vi "Periodic Tasks.vi"(8 "error in":errorcluster) -> ()   [LabVIEW 2018]
doc: "This VI runs in parallel to other tasks. It can contain as many user-defined periodic loops as you need. These can carry out PID or other sorts of timed response."
uses:
  <vilib>/Rock Robotics/WPI/ThirdParty/Phoenix-LabVIEW/Motor Controller/Controls/CTRE_Phoenix_MotorControl_ControlMode.ctl
  <vilib>/Rock Robotics/WPI/Utilities/WPI_GetSetVariantRefNum.vi
  <vilib>/Rock Robotics/Network Tables/NT Write Boolean Array.vi
  <vilib>/Rock Robotics/Network Tables/NT Write Numeric Array.vi
  <vilib>/Rock Robotics/Network Tables/NT Write Boolean.vi
  <vilib>/Rock Robotics/WPI/RobotDrive/WPI_RobotDriveMecanumDrive_Cartesian.vi
  <vilib>/Rock Robotics/WPI/ThirdParty/Phoenix-LabVIEW/Motor Controller/Get/CTRE_Phoenix_MotorController_GetAnalogData.vi
  <vilib>/Rock Robotics/Network Tables/NT Write Number.vi
panel:
  in  "Jack speed 3-2":dbl=-1.0
  in  "Jack drive 1-2":dbl=-0.75
  in  "Jack speed 2-2":dbl=1.0
  in  "Jack speed 1-2":dbl=1.0
  in  "Arm speed-2":dbl=-0.41
  in  "Pre Climb 2":i32=146
  in  "Load Cargo":i32=385
  in  "Arm speed":dbl=-0.55
  in  "Jack speed 1":dbl=1.0
  in  "Jack speed 2":dbl=1.0
  in  "Jack drive 1":dbl=-0.75
  in  "Jack speed 3":dbl=-1.0
  in  "Pre Climb":i32=80
  in  "Release Time":i32=7
  in  "Grab Drive Time":i32=7
  in  "Grab Wait Time":i32=2
  in  "Grab Time":i32=5
  in  "Home":i32=70
  in  "C High":i32=890
  in  "C Med":i32=540
  in  "C Low":i32=230
  in  "H High":i32=809
  in  "H Med":i32=475
  in  "H Low":i32=140
  out "Jack PO":dbl=-0.007874015748031496
  out "Arm PO":dbl=-0.007874015748031496
  out "Arm position":i32=145
  # "Climb 2 Case Values"
  # "Arm Actuators"
  # "Jack Mech."
  # "Jack Wheels"
  # "In pre climb cases add about 5% drive forward"
  # "Climb Case Values"
  # "Arm Actuators"
  # "Jack Mech."
  # "Jack Wheels"
  # "Grab and Release Times and Values\n                 In State Machine"
  # "State Machine Values for Positions"
  # "Proto Values Before Heartland"
  # "Pre Climb 2 146"
  # "H Low 171\nH Med 475\nH High 809"
  # "C Low 230\nC Med 540\nC High 890"
  # "Load Cargo 385\nHome 70\nPre Climb 80"
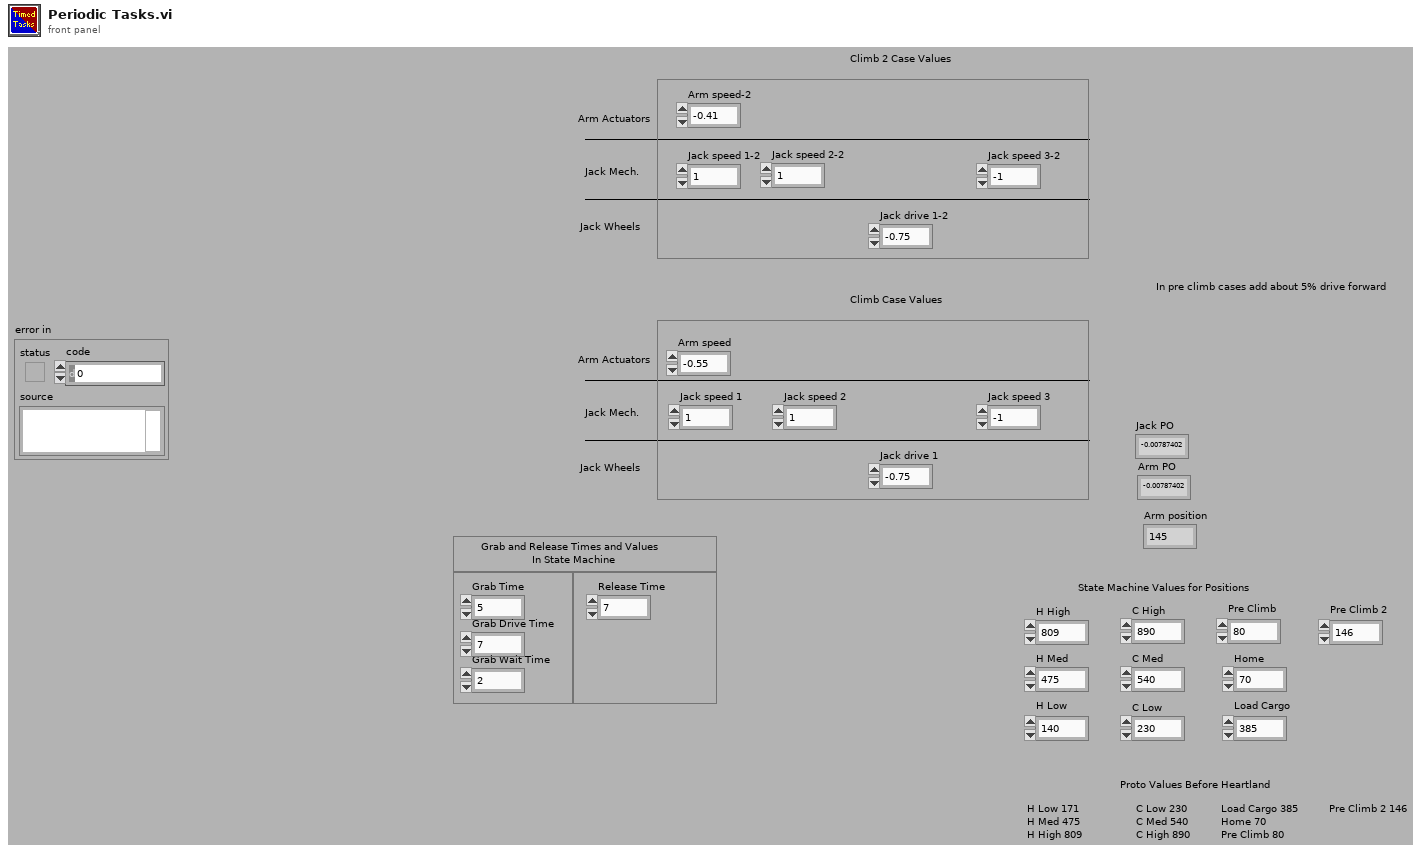
[diagram p1: front panel]
types:
  T1 = enum16{"Wait", "H.Low", "H.Med", "H.High", "C.Low", "C.Med", "C.High", "Home", "Pull Out Grab", "Pull Out Release", "Pre Climb", "Upward Travel", "Extra Jack Time", "Forward Travel", "Jack Retrieval", "Load Cargo", "Pre Climb 2", "Upward Travel 2", "Extra Jack Time 2", "Forward Travel 2", "Jack Retrieval 2"}
  T2 = typedef "WPI_MotorControlDeviceRef.ctl" = cluster{"DeviceStatus":errorcluster, "Type":T3, "PWM":cluster{"PWM Channel":T4, "DeadBand":T5}, "CAN":cluster{"Device Number":u8, "SetOutput VI Ref":variant, "GetOutput VI Ref":variant, "Enable VI Ref":variant, "Disable VI Ref":variant, "Data":variant}, "Invert":bool, "DIO PWM":cluster{"PWM \"Enable\" Channel":T4, "DIOChannel":T6, "PWM Rate":dbl}}
  T3 = typedef "WPI_MotorControlType.ctl" = enum16{"PWM", "CAN", "DIO PWM"}
  T4 = typedef "FPGA_DIOPWMChannel.ctl" = enum8{"PWM 0", "PWM 1", "PWM 2", "PWM 3", "PWM 4", "PWM 5", "PWM 6", "PWM 7", "PWM 8", "PWM 9", "PWM MXP 0", "PWM MXP 1", "PWM MXP 2", "PWM MXP 3", "PWM MXP 4", "PWM MXP 5", "PWM MXP 6", "PWM MXP 7", "PWM MXP 8", "PWM MXP 9", "Invalid"}
  T5 = typedef "WPI_PWMDeadband.ctl" = cluster{"Name":string, "maxPositivePwm":i32, "minPositivePwm":i32, "centerPwm":i32, "maxNegativePwm":i32, "minNegativePwm":i32, "angularRange":u16}
  T6 = typedef "FPGA_DIOChannel.ctl" = enum8{"DIO 0", "DIO 1", "DIO 2", "DIO 3", "DIO 4", "DIO 5", "DIO 6", "DIO 7", "DIO 8", "DIO 9", "DIO MXP 0", "DIO MXP 1", "DIO MXP 2", "DIO MXP 3", "DIO MXP 4", "DIO MXP 5", "DIO MXP 6", "DIO MXP 7", "DIO MXP 8", "DIO MXP 9", "DIO MXP 10", "DIO MXP 11", "DIO MXP 12", "DIO MXP 13", "DIO MXP 14", "DIO MXP 15", "SPI Port CS1", "SPI Port CS2", "SPI Port CS3", "SPI Port MISO", "SPI Port MOSI", "Invalid"}
  T7 = typedef "WPI_JoystickDevRef.ctl" = cluster{"Device":T8}
  T8 = typedef "WPI_JoystickDeviceEnum.ctl" = enum16{"USB 0", "USB 1", "USB 2", "USB 3", "USB 4", "USB 5"}
  T9 = typedef "CTRE_Phoenix_MotorControl_ControlMode.ctl" = u16
  T10 = typedef "WPI_RobotDriveDevRef.ctl" = cluster{"DevStatus":errorcluster, "Motors[]":T2[], "Square Inputs":bool, "Max Output":dbl}
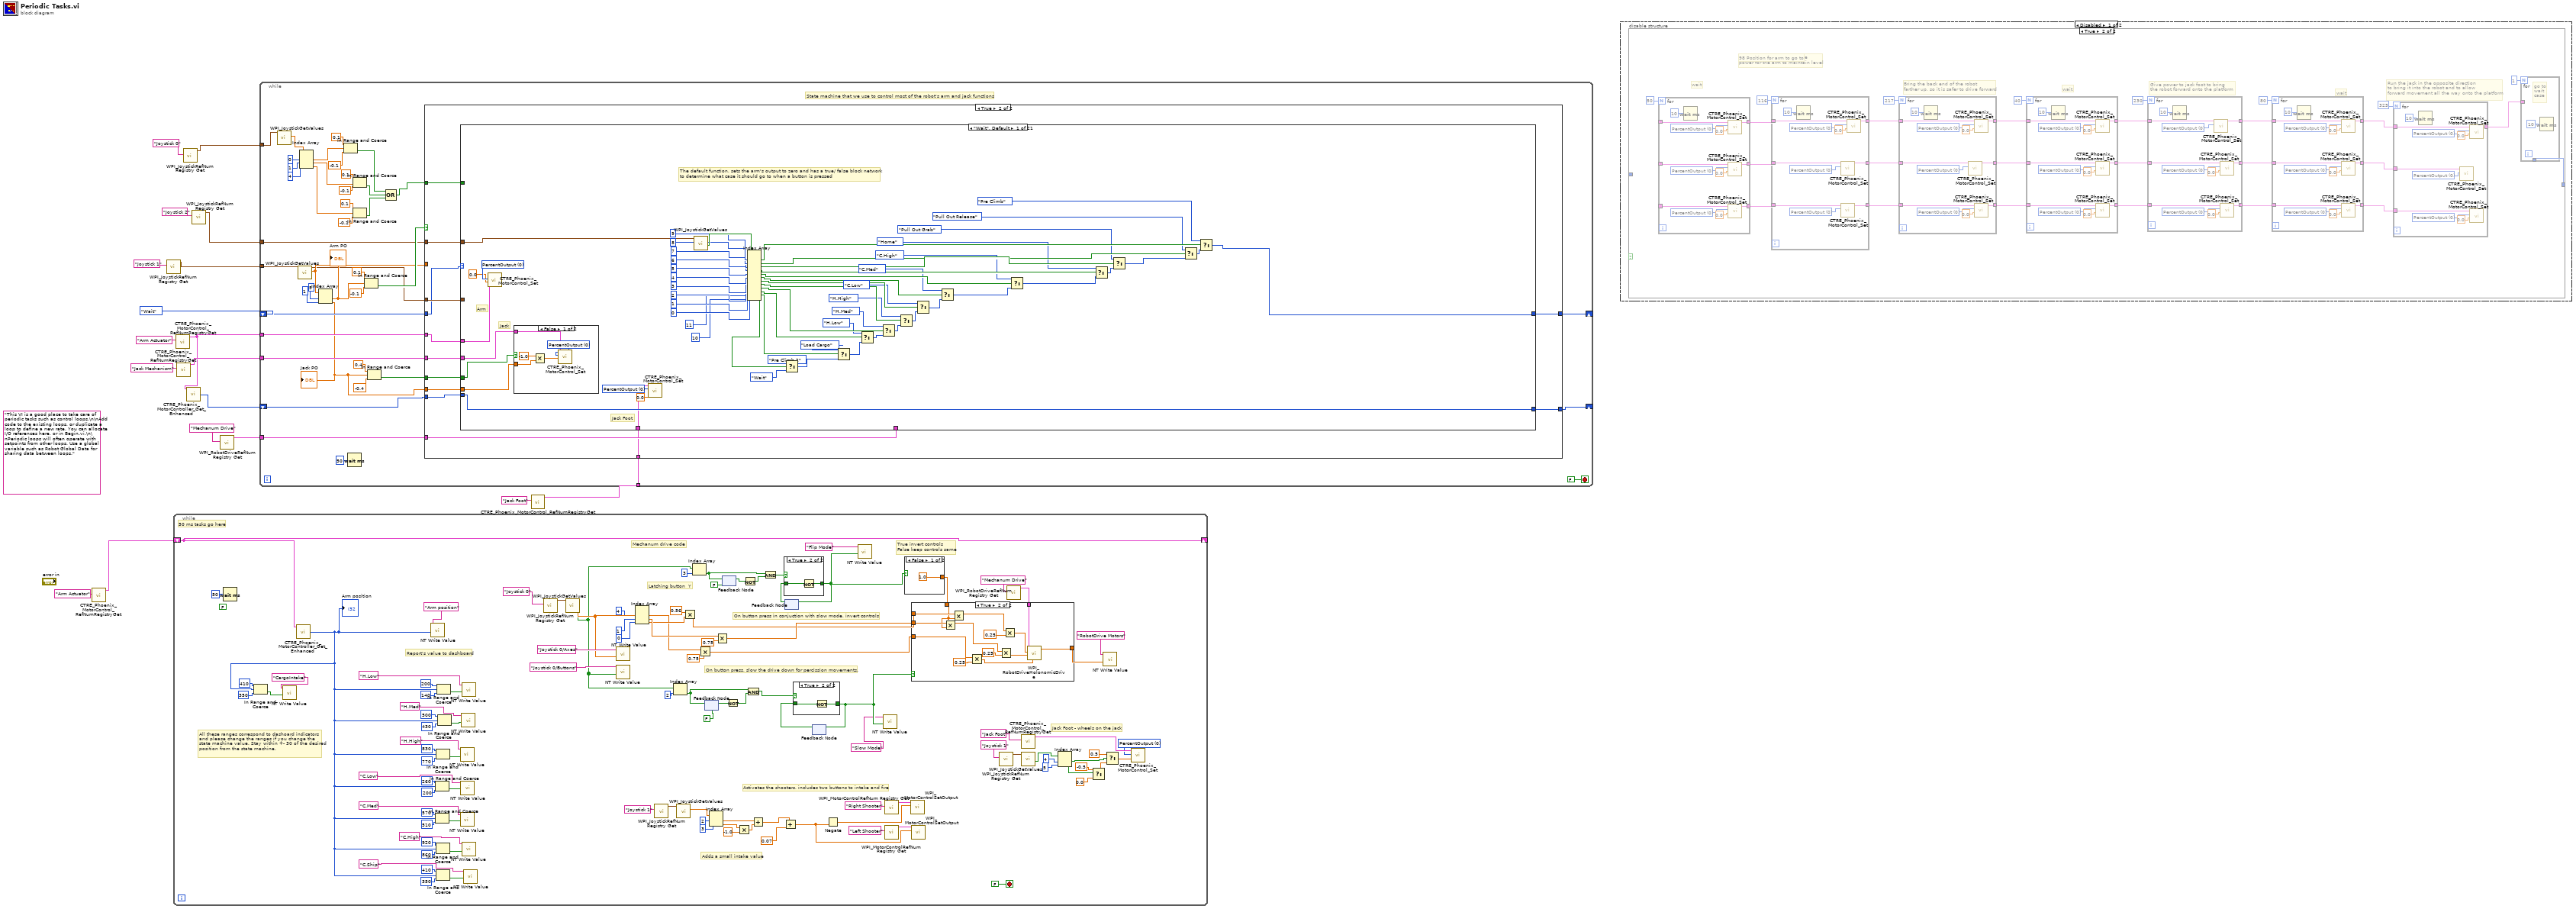
[diagram p0: block diagram]
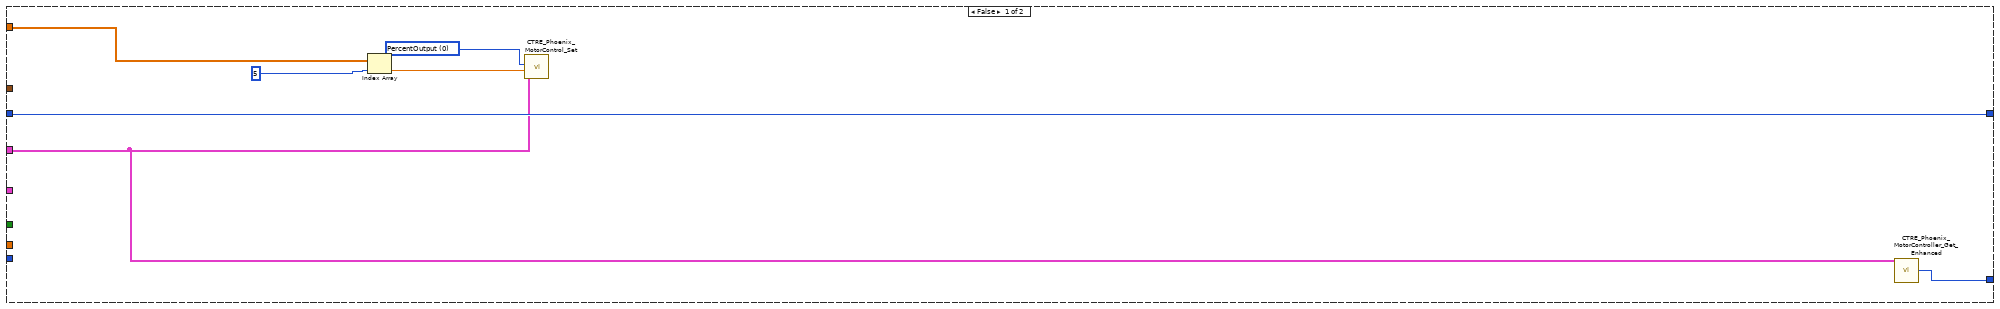
[diagram p4: hidden frame]
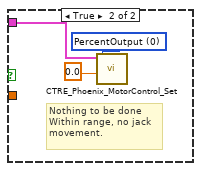
[diagram p5: hidden frame]
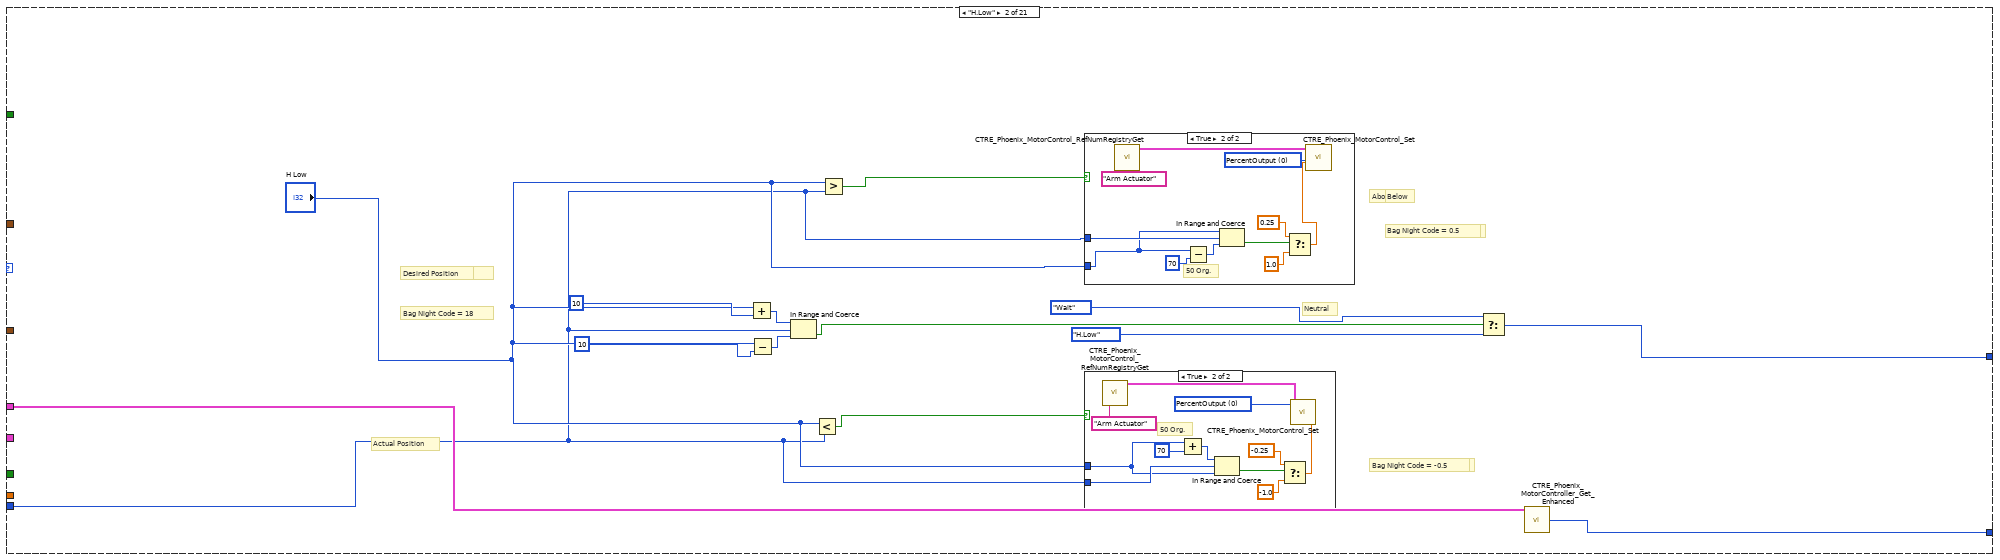
[diagram p6: hidden frame]
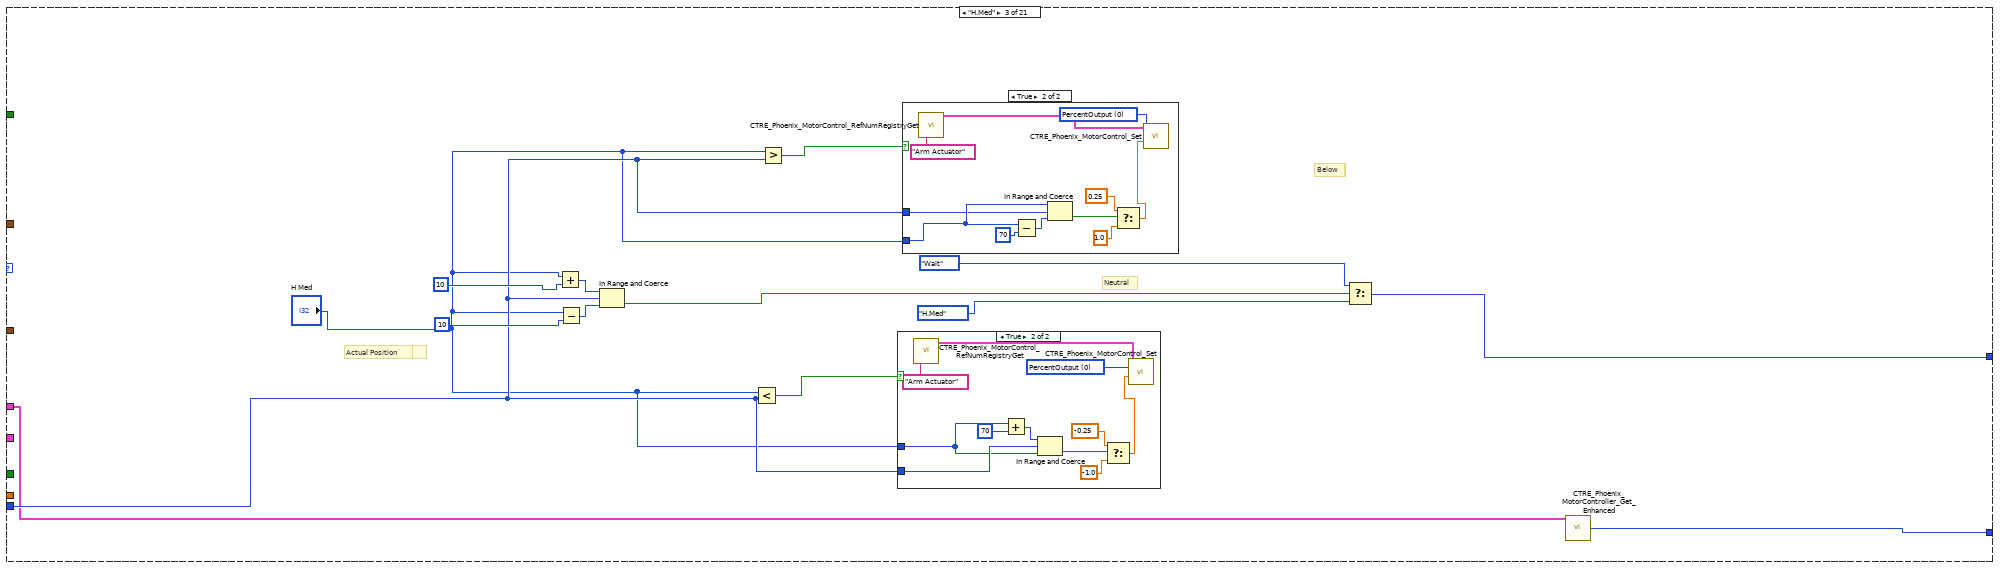
[diagram p9: hidden frame]
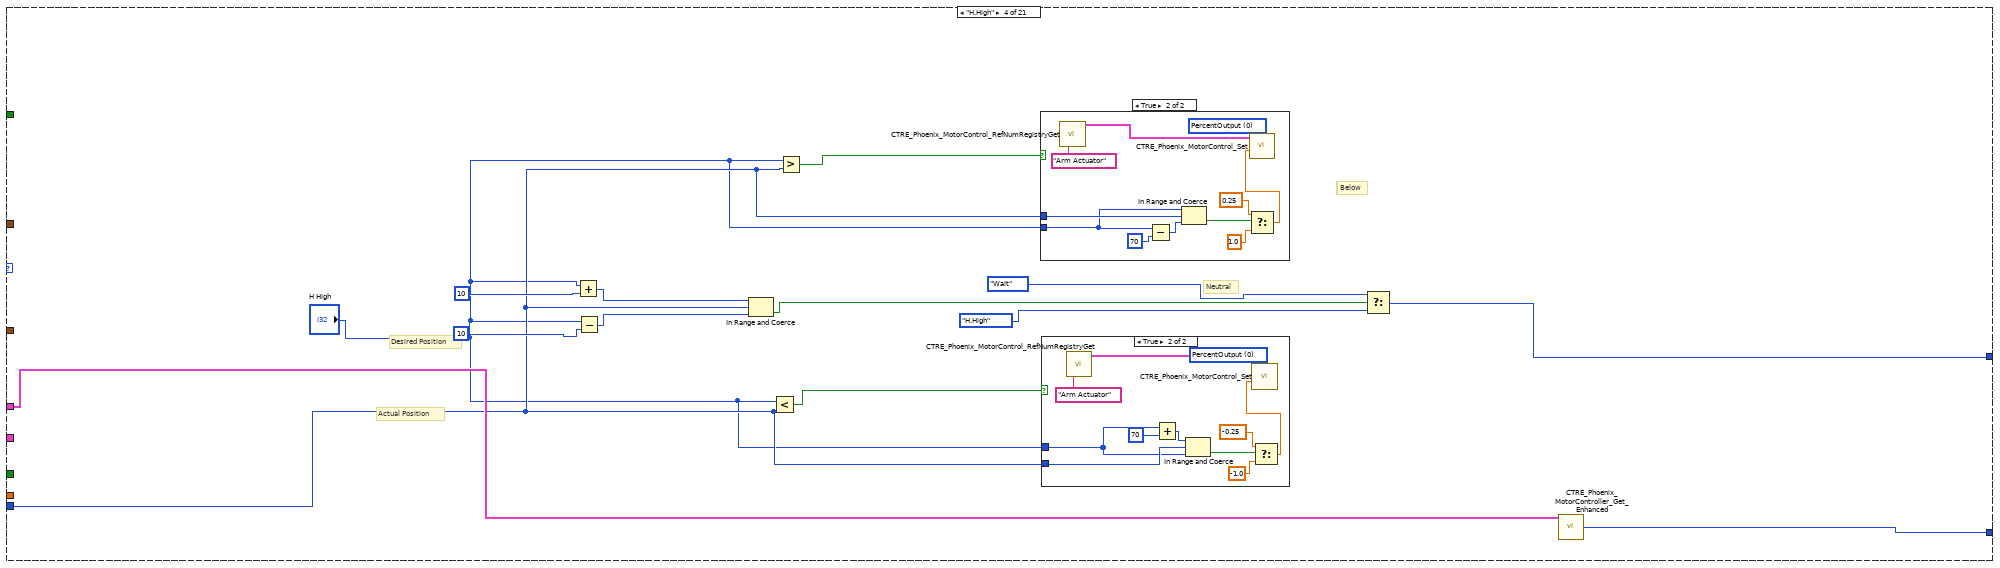
[diagram p12: hidden frame]
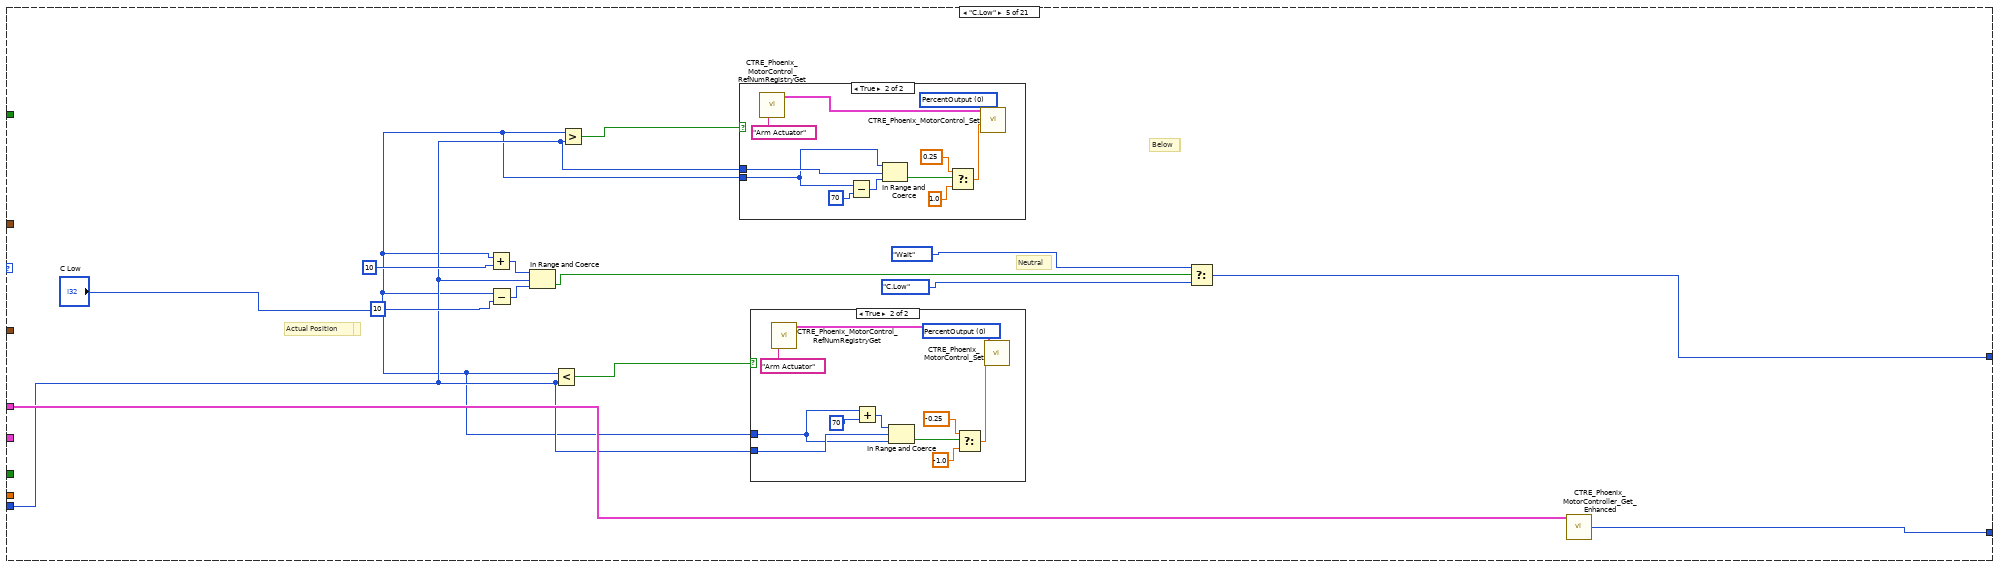
[diagram p15: hidden frame]
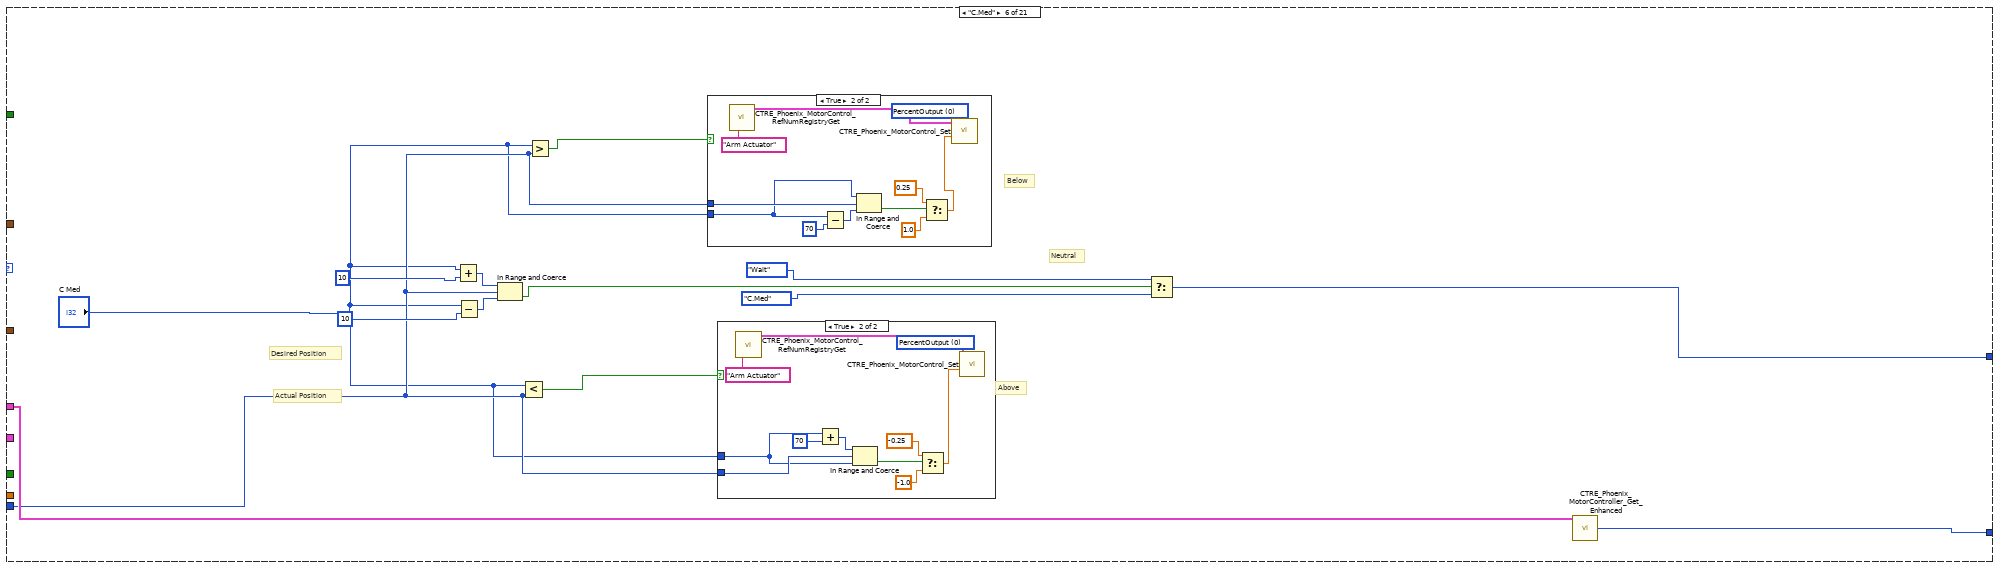
[diagram p18: hidden frame]
diagram:
  (unwired) "This VI is a good place to take care of periodic tasks such as control loops.\n\nAdd code to the existing loops, or duplicate a loop to define a new rate. You can allocate I/O references here, or in Begin.vi.\n\nPeriodic loops will often operate with setpoints from other loops. Use a global variable such as Robot Global Data for sharing data between loops."
  n1 = call <vilib>:"CTRE_Phoenix_MotorControl_RefNumRegistryGet.vi"("refnum name"="Arm Actuator") -> ("PhoenixMotorControlDevRef"=w17:T2)  [unwired: 9 in, 1 out]
  n2 = call <vilib>:"WPI_JoystickRefNum Registry Get.vi"("refnum name"="Joystick 1") -> ("JoystickDevRef"=w13:T7)  [unwired: 9 in, 1 out]
  n3 = while {
    shift-right: [w53] -> _
    shift-left: w17 -> [w53]
    stop <- FALSE stop-if-true
    w30 = T9 0 items=["PercentOutput"=0, "Position"=1, "Velocity"=2, "Current"=3, "Follower"=5, "MotionProfile"=6, "MotionMagic"=7, "MotionProfileArc"=10, "Disabled"=15] ("Control Mode")
    (unwired) FALSE
    # "On button press in conjuction with slow mode, invert controls"
    # "Latching button  Y"
    # "True invert controls\nFalse keep controls same"
    # "Jack Foot - wheels on the jack"
    # "All these ranges correspond to dashoard indicators\nand please change the ranges if you change the \nstate machine value. Stay within +- 30 of the desired\nposition from the state machine."
    # "Adds a small intake value"
    # "On button press, slow the drive down for percission movements."
    # "Report's value to dashboard"
    # "Mechanum drive code"
    # "Activates the shooters, includes two buttons to intake and fire"
    # "50 ms tasks go here"
    n4 = Wait (ms)(milliseconds to wait=u32 50) -> ()  [unwired: 1 out]
    n5 = call-poly <vilib>:"CTRE_Phoenix_MotorController_Get_Enhanced.vi"("PhoenixMotorControlDevRef"=w53) -> ("AnalogInRaw"=w62:i32)  [unwired: 10 in, 4 out]
    "Arm position" <- w62
    n6 = In Range and Coerce(upper limit=410, x=w62, lower limit=350) -> (In Range?=w59:bool)  [unwired: 1 out]
    n7 = call-poly <vilib>:"NT Write Value.vi"("Boolean"=w59, "Name"="CargoIntake") -> ()  [unwired: 9 in, 1 out]
    n8 = call-poly <vilib>:"NT Write Value.vi"("Numeric"=w62, "Name"="Arm position") -> ()  [unwired: 9 in, 1 out]
    n9 = In Range and Coerce(upper limit=570, x=w62, lower limit=510) -> (In Range?=w79:bool)  [unwired: 1 out]
    n10 = In Range and Coerce(upper limit=260, x=w62, lower limit=200) -> (In Range?=w78:bool)  [unwired: 1 out]
    n11 = In Range and Coerce(upper limit=830, x=w62, lower limit=770) -> (In Range?=w77:bool)  [unwired: 1 out]
    n12 = In Range and Coerce(upper limit=920, x=w62, lower limit=860) -> (In Range?=w81:bool)  [unwired: 1 out]
    n13 = In Range and Coerce(upper limit=410, x=w62, lower limit=350) -> (In Range?=w80:bool)  [unwired: 1 out]
    n14 = In Range and Coerce(upper limit=200, x=w62, lower limit=140) -> (In Range?=w75:bool)  [unwired: 1 out]
    n15 = In Range and Coerce(upper limit=500, x=w62, lower limit=430) -> (In Range?=w76:bool)  [unwired: 1 out]
    n16 = call-poly <vilib>:"NT Write Value.vi"("Boolean"=w77, "Name"="H.High") -> ()  [unwired: 9 in, 1 out]
    n17 = call-poly <vilib>:"NT Write Value.vi"("Boolean"=w79, "Name"="C.Med") -> ()  [unwired: 9 in, 1 out]
    n18 = call-poly <vilib>:"NT Write Value.vi"("Boolean"=w78, "Name"="C.Low") -> ()  [unwired: 9 in, 1 out]
    n19 = call-poly <vilib>:"NT Write Value.vi"("Boolean"=w76, "Name"="H.Med") -> ()  [unwired: 9 in, 1 out]
    n20 = call-poly <vilib>:"NT Write Value.vi"("Boolean"=w75, "Name"="H.Low") -> ()  [unwired: 9 in, 1 out]
    n21 = call-poly <vilib>:"NT Write Value.vi"("Boolean"=w81, "Name"="C.High") -> ()  [unwired: 9 in, 1 out]
    n22 = call-poly <vilib>:"NT Write Value.vi"("Boolean"=w80, "Name"="C.Ship") -> ()  [unwired: 9 in, 1 out]
    n23 = call <vilib>:"WPI_JoystickRefNum Registry Get.vi"("refnum name"="Joystick 0") -> ("JoystickDevRef"=w126:T7)  [unwired: 1 in, 9 out]
    n24 = call <vilib>:"WPI_JoystickGetValues.vi"("JoystickDevRef"=w126) -> ("Buttons"=w20:bool[], "Axes"=w123:dbl[])  [unwired: 6 in, 3 out]
    n25 = call-poly <vilib>:"NT Write Value.vi"("Numeric Array"=w123, "Name"="Joystick 0/Axes") -> ()  [unwired: 9 in, 1 out]
    n26 = call-poly <vilib>:"NT Write Value.vi"("Boolean Array"=w20, "Name"="Joystick 0/Buttons") -> ()  [unwired: 9 in, 1 out]
    n27 = Index Array(array=w123, index #1=4 ("index"), index #2=1 ("index"), index #3=0 ("index")) -> (element #1=w54:dbl, element #2=w105:dbl, element #3=w55:dbl)
    n28 = call <vilib>:"WPI_JoystickRefNum Registry Get.vi"("refnum name"="Joystick 1") -> ("JoystickDevRef"=w122:T7)  [unwired: 1 in, 9 out]
    n29 = Index Array(array=w20, index=2) -> (element=w49:bool)
    n30 = call <vilib>:"WPI_JoystickGetValues.vi"("JoystickDevRef"=w122) -> ("Axes"=w116:dbl[])  [unwired: 6 in, 4 out]
    n31 = Multiply(x=0.56, y=w55) -> (x*y=w56:dbl)
    n32 = Index Array(array=w20, index=3) -> (element=w24:bool)
    n33 = Multiply(x=w54, y=0.75) -> (x*y=w66:dbl)
    n34 = feedback-in #1(w49) -> ()
    n35 = feedback #1(FALSE) -> (w51:bool)
    n36 = Index Array(array=w116, index #1=2 ("index"), index #2=3 ("index")) -> (element #1=w110:dbl, element #2=w112:dbl)
    n37 = Multiply(x=w105, y=0.75) -> (x*y=w67:dbl)
    n38 = feedback #2(FALSE) -> (w26:bool)
    n39 = feedback-in #2(w24) -> ()
    n40 = Not(x=w51) -> (.not. x?=w50:bool)
    n41 = Multiply(x=w112, y=-1.0) -> (x*y=w111:dbl)
    n42 = Not(x=w26) -> (.not. x?=w25:bool)
    n43 = And(x=w49, y=w50) -> (x .and. y?=w48:bool)
    n44 = Add(x=w110, y=w111) -> (x+y=w99:dbl)
    n45 = And(x=w24, y=w25) -> (x .and. y?=w23:bool)
    n46 = Add(x=w99, y=0.07) -> (x+y=w97:dbl)
    n47 = feedback #3() -> (w22:bool)  [unwired: 1 in]
    n48 = case shown="True" w23 {
      tunnel: w22 -> [w129 w131]
      tunnel: [w129 w130] -> w19
      frame False {
      }
      frame True {
        n49 = Not(x=w131) -> (.not. x?=w130:bool)
      }
    }
    n50 = feedback-in #3(w19) -> ()
    n51 = feedback #4() -> (w47:bool)  [unwired: 1 in]
    n52 = case shown="True" w48 {
      tunnel: w47 -> [w134 w136]
      tunnel: [w134 w135] -> w46
      frame False {
      }
      frame True {
        n53 = Not(x=w136) -> (.not. x?=w135:bool)
      }
    }
    n54 = feedback-in #4(w46) -> ()
    n55 = Negate(x=w97) -> (-x=w109:dbl)
    n56 = call-poly <vilib>:"NT Write Value.vi"("Boolean"=w19, "Name"="Flip Mode") -> ()  [unwired: 9 in, 1 out]
    n57 = call-poly <vilib>:"NT Write Value.vi"("Boolean"=w46, "Name"="Slow Mode") -> ()  [unwired: 9 in, 1 out]
    n58 = call <vilib>:"WPI_MotorControlRefNum Registry Get.vi"("refnum name"="Right Shooter") -> ("MotorControlDevRef"=w118:T2)  [unwired: 9 in, 1 out]
    n59 = call <vilib>:"WPI_MotorControlRefNum Registry Get.vi"("refnum name"="Left Shooter") -> ("MotorControlDevRef"=w117:T2)  [unwired: 9 in, 1 out]
    n60 = case shown="False" w19 {
      tunnel: [1.0 -1.0] -> w29
      frame False {
      }
      frame True {
      }
    }
    n61 = call <vilib>:"WPI_MotorControlSetOutput.vi"("Output"=w109, "MotorControlDevRef"=w118) -> ()  [unwired: 7 in, 3 out]
    n62 = call <vilib>:"WPI_MotorControlSetOutput.vi"("Output"=w97, "MotorControlDevRef"=w117) -> ()  [unwired: 7 in, 3 out]
    n63 = call <vilib>:"WPI_JoystickRefNum Registry Get.vi"("refnum name"="Joystick 1") -> ("JoystickDevRef"=w43:T7)  [unwired: 1 in, 9 out]
    n64 = call <vilib>:"WPI_RobotDriveRefNum Registry Get.vi"("refnum name"="Mechanum Drive") -> ("RobotDriveDevRef"=w106:T10)  [unwired: 1 in, 9 out]
    n65 = case shown="True" w46 {
      tunnel: w106 -> [w139 w155]
      tunnel: [w140 w154] -> w104
      tunnel: w56 -> [w137 w146]
      tunnel: w67 -> [w141 w149]
      tunnel: w66 -> [w138 w142]
      tunnel: w29 -> [_ w143]
      frame False {
        n66 = call-poly <vilib>:"WPI_RobotDriveHolonomicDrive.vi"("Rotation"=w138, "Y"=w141, "X"=w137, "RobotDriveDevRef"=w139) -> ("Motor Values"=w140:dbl[])  [unwired: 5 in, 2 out]
      }
      frame True {
        n67 = Multiply(x=w149, y=w143) -> (x*y=w145:dbl)
        n68 = Multiply(x=w146, y=w143) -> (x*y=w144:dbl)
        n69 = Multiply(x=w142, y=0.25 ("x")) -> (x*y=w153:dbl)
        n70 = Multiply(x=w145, y=0.25) -> (x*y=w151:dbl)
        n71 = Multiply(x=w144, y=0.25 ("x")) -> (x*y=w148:dbl)
        n72 = call-poly <vilib>:"WPI_RobotDriveHolonomicDrive.vi"("Rotation"=w153, "Y"=w151, "X"=w148, "RobotDriveDevRef"=w155) -> ("Motor Values"=w154:dbl[])  [unwired: 5 in, 2 out]
      }
    }
    n73 = call <vilib>:"WPI_JoystickGetValues.vi"("JoystickDevRef"=w43) -> ("Buttons"=w40:bool[])  [unwired: 6 in, 4 out]
    n74 = call <vilib>:"CTRE_Phoenix_MotorControl_RefNumRegistryGet.vi"("refnum name"="Jack Foot") -> ("PhoenixMotorControlDevRef"=w33:T2)  [unwired: 9 in, 1 out]
    n75 = Index Array(array=w40, index #1=4 ("index"), index #2=5 ("index")) -> (element #1=w38:bool, element #2=w39:bool)
    n76 = Select(t=-0.5, s=w39, f=0.0) -> (s? t:f=w37:dbl)
    n77 = call-poly <vilib>:"NT Write Value.vi"("Numeric Array"=w104, "Name"="RobotDrive Motors") -> ()  [unwired: 9 in, 1 out]
    n78 = Select(t=0.5, s=w38, f=w37) -> (s? t:f=w31:dbl)
    n79 = call <vilib>:"CTRE_Phoenix_MotorControl_Set.vi"("Output"=w31, "Control Mode"=w30, "PhoenixMotorControlDevRef"=w33) -> ()  [unwired: 7 in, 2 out]
  }
  n80 = call <vilib>:"CTRE_Phoenix_MotorControl_RefNumRegistryGet.vi"("refnum name"="Arm Actuator") -> ("PhoenixMotorControlDevRef"=w6:T2)  [unwired: 9 in, 1 out]
  n81 = call <vilib>:"CTRE_Phoenix_MotorControl_RefNumRegistryGet.vi"("refnum name"="Jack Mechanism") -> ("PhoenixMotorControlDevRef"=w9:T2)  [unwired: 9 in, 1 out]
  n82 = call <vilib>:"WPI_JoystickRefNum Registry Get.vi"("refnum name"="Joystick 0") -> ("JoystickDevRef"=w11:T7)  [unwired: 9 in, 1 out]
  n83 = call-poly <vilib>:"CTRE_Phoenix_MotorController_Get_Enhanced.vi"("PhoenixMotorControlDevRef"=w6) -> ("AnalogInRaw"=w3:i32)  [unwired: 10 in, 4 out]
  n84 = call <vilib>:"WPI_JoystickRefNum Registry Get.vi"("refnum name"="Joystick 2") -> ("JoystickDevRef"=w4:T7)  [unwired: 9 in, 1 out]
  n85 = call <vilib>:"WPI_RobotDriveRefNum Registry Get.vi"("refnum name"="Mechanum Drive") -> ("RobotDriveDevRef"=w7:T10)  [unwired: 1 in, 9 out]
  n86 = call <vilib>:"CTRE_Phoenix_MotorControl_RefNumRegistryGet.vi"("refnum name"="Jack Foot") -> ("PhoenixMotorControlDevRef"=w1:T2)  [unwired: 9 in, 1 out]
  n87 = while {
    shift-right: [w173] -> _
    shift-left: T1."Wait" -> [w157]
    tunnel: w13 -> [w196]
    tunnel: w6 -> [w191]
    tunnel: w11 -> [w174]
    tunnel: w9 -> [w168]
    tunnel: w7 -> [w167]
    tunnel: w4 -> [w166]
    shift-right: [w164] -> _
    shift-left: w3 -> [w165]
    tunnel: w1 -> [w159]
    stop <- FALSE stop-if-true
    # "State machine that we use to control most of the robot's arm and jack functions"
    n88 = call <vilib>:"WPI_JoystickGetValues.vi"("JoystickDevRef"=w174) -> ("Axes"=w183:dbl[])  [unwired: 6 in, 4 out]
    n89 = call <vilib>:"WPI_JoystickGetValues.vi"("JoystickDevRef"=w196) -> ("Axes"=w190:dbl[], "JoystickDevRef"=w189:T7)  [unwired: 6 in, 3 out]
    n90 = Index Array(array=w183, index #1=0 ("index"), index #2=1 ("index"), index #3=4 ("index")) -> (element #1=w184:dbl, element #2=w176:dbl, element #3=w175:dbl)
    n91 = Index Array(array=w190, index #1=5 ("index"), index #2=1 ("index")) -> (element #1=w193:dbl, element #2=w156:dbl)
    "Jack PO" <- w156
    "Arm PO" <- w193
    n92 = In Range and Coerce(upper limit=0.1, x=w184, lower limit=-0.1) -> (In Range?=w161:bool)  [unwired: 1 out]
    n93 = Wait (ms)(milliseconds to wait=u32 50) -> ()  [unwired: 1 out]
    n94 = In Range and Coerce(upper limit=0.1, x=w176, lower limit=-0.1) -> (In Range?=w163:bool)  [unwired: 1 out]
    n95 = In Range and Coerce(upper limit=0.1, x=w175, lower limit=-0.1) -> (In Range?=w162:bool)  [unwired: 1 out]
    n96 = In Range and Coerce(upper limit=0.1, x=w193, lower limit=-0.1) -> (In Range?=w192:bool)  [unwired: 1 out]
    n97 = In Range and Coerce(upper limit=0.4, x=w156, lower limit=-0.4) -> (In Range?=w169:bool)  [unwired: 1 out]
    n98 = Compound Arithmetic op=OR(w161, w163, w162) -> (w160:bool)
    n99 = case shown="True" w192 {
      tunnel: w157 -> [w200 w206]
      tunnel: w191 -> [w198 w217]
      tunnel: w190 -> [w201 _]
      tunnel: w189 -> [_ w216]
      tunnel: w160 -> [_ w215]
      tunnel: [w200 w214] -> w173
      tunnel: w169 -> [_ w213]
      tunnel: w168 -> [_ w212]
      tunnel: w167 -> [_ w211]
      tunnel: w165 -> [_ w209]
      tunnel: w166 -> [_ w210]
      tunnel: [w199 w208] -> w164
      tunnel: w159 -> [_ w207]
      tunnel: w156 -> [_ w205]
      frame False {
        w204 = T9 0 items=["PercentOutput"=0, "Position"=1, "Velocity"=2, "Current"=3, "Follower"=5, "MotionProfile"=6, "MotionMagic"=7, "MotionProfileArc"=10, "Disabled"=15] ("Control Mode")
        n100 = Index Array(array=w201, index=5) -> (element=w202:dbl)
        n101 = call <vilib>:"CTRE_Phoenix_MotorControl_Set.vi"("Output"=w202, "Control Mode"=w204, "PhoenixMotorControlDevRef"=w198) -> ()  [unwired: 7 in, 2 out]
        n102 = call-poly <vilib>:"CTRE_Phoenix_MotorController_Get_Enhanced.vi"("PhoenixMotorControlDevRef"=w198) -> ("AnalogInRaw"=w199:i32)  [unwired: 10 in, 4 out]
      }
      frame True {
        n103 = case shown="\"Wait\", Default" w206 {
          selector: w206 -> [_ _ _ _ _ _ _ _ w543 w570 _ _ _ _ _ _ _ _ _ _ _]
          tunnel: w217 -> [w278 w291 w325 w363 w399 w435 w471 w507 w539 w565 w592 w631 w653 w675 w697 w717 w750 w791 w813 w836 w862]
          tunnel: w216 -> [_ _ _ _ _ _ _ _ _ _ _ _ _ _ _ _ _ _ _ _ _]
          tunnel: w215 -> [_ _ _ _ _ _ _ _ w544 w569 _ _ _ _ _ _ _ _ _ _ _]
          tunnel: [w242 w293 w329 w366 w401 w437 w475 w509 w542 w568 w590 w625 w647 w670 w692 w715 w749 w784 w807 w830 w856] -> w214
          tunnel: w213 -> [w218 _ _ _ _ _ _ _ _ _ _ _ _ _ _ _ _ _ _ _ _]
          tunnel: w212 -> [w220 _ _ _ _ _ _ _ _ _ _ w628 w652 w674 w696 _ _ w790 w812 w835 w861]
          tunnel: w211 -> [_ _ _ _ _ _ _ _ w541 w567 _ _ _ _ _ _ _ _ _ w829 _]
          tunnel: w209 -> [w244 w289 w327 w362 w398 w434 w470 w506 _ _ w591 w632 w654 w676 w698 w716 w751 w793 w815 w838 w864]
          tunnel: w210 -> [w266 _ _ _ _ _ _ _ _ _ _ _ _ _ _ _ _ _ _ _ _]
          tunnel: [w244 w292 w328 w364 w400 w436 w472 w508 w540 w566 w589 w632 w654 w676 w698 w714 w748 w793 w815 w838 w864] -> w208
          tunnel: w207 -> [w223 _ _ _ _ _ _ _ _ _ _ w627 w651 w673 w695 _ _ w789 w811 w834 w860]
          tunnel: w205 -> [w219 _ _ _ _ _ _ _ _ _ _ _ _ _ _ _ _ _ _ _ _]
          frame "Wait", Default {
            w222 = T9 0 items=["PercentOutput"=0, "Position"=1, "Velocity"=2, "Current"=3, "Follower"=5, "MotionProfile"=6, "MotionMagic"=7, "MotionProfileArc"=10, "Disabled"=15] ("Control Mode")
            w277 = T9 0 items=["PercentOutput"=0, "Position"=1, "Velocity"=2, "Current"=3, "Follower"=5, "MotionProfile"=6, "MotionMagic"=7, "MotionProfileArc"=10, "Disabled"=15] ("Control Mode")
            # "Jack Foot"
            # "Jack"
            # "Arm"
            # "The default function, sets the arm's output to zero and has a true/ false block network\nto determine what case it should go to when a button is pressed"
            n104 = call <vilib>:"CTRE_Phoenix_MotorControl_Set.vi"("Output"=0.0, "Control Mode"=w277, "PhoenixMotorControlDevRef"=w278) -> ()  [unwired: 7 in, 2 out]
            n105 = case shown="False" w218 {
              tunnel: w220 -> [w279 w286]
              tunnel: w219 -> [w280 _]
              frame False {
                w281 = T9 0 items=["PercentOutput"=0, "Position"=1, "Velocity"=2, "Current"=3, "Follower"=5, "MotionProfile"=6, "MotionMagic"=7, "MotionProfileArc"=10, "Disabled"=15] ("Control Mode")
                n106 = Multiply(x=-1.0, y=w280) -> (x*y=w283:dbl)
                n107 = call <vilib>:"CTRE_Phoenix_MotorControl_Set.vi"("Output"=w283, "Control Mode"=w281, "PhoenixMotorControlDevRef"=w279) -> ()  [unwired: 7 in, 2 out]
              }
              frame True {
                w285 = T9 0 items=["PercentOutput"=0, "Position"=1, "Velocity"=2, "Current"=3, "Follower"=5, "MotionProfile"=6, "MotionMagic"=7, "MotionProfileArc"=10, "Disabled"=15] ("Control Mode")
                # "Nothing to be done\nWithin range, no jack\nmovement."
                n108 = call <vilib>:"CTRE_Phoenix_MotorControl_Set.vi"("Output"=0.0 ("x"), "Control Mode"=w285, "PhoenixMotorControlDevRef"=w286) -> ()  [unwired: 7 in, 2 out]
              }
            }
            n109 = call <vilib>:"CTRE_Phoenix_MotorControl_Set.vi"("Output"=0.0, "Control Mode"=w222, "PhoenixMotorControlDevRef"=w223) -> ()  [unwired: 7 in, 2 out]
            n110 = call <vilib>:"WPI_JoystickGetValues.vi"("JoystickDevRef"=w266) -> ("Buttons"=w265:bool[])  [unwired: 6 in, 4 out]
            n111 = Index Array(array=w265, index #1=9 ("index"), index #2=8 ("index"), index #3=7 ("index"), index #4=6 ("index"), index #5=5 ("index"), index #6=4 ("index"), index #7=3 ("index"), index #8=2 ("index"), index #9=1 ("index"), index #10=0 ("index"), index #11=11 ("index"), index #12=10 ("index")) -> (element #1=w255:bool, element #2=w256:bool, element #3=w257:bool, element #4=w258:bool, element #5=w259:bool, element #6=w260:bool, element #7=w261:bool, element #8=w262:bool, element #9=w263:bool, element #10=w264:bool, element #11=w240:bool, element #12=w238:bool)
            n112 = Select(t=T1."Pre Climb 2", s=w238, f=T1."Wait") -> (s? t:f=w239:T1)
            n113 = Select(t=T1."Load Cargo", s=w240, f=w239) -> (s? t:f=w241:T1)
            n114 = Select(t=T1."H.Low", s=w264, f=w241) -> (s? t:f=w275:T1)
            n115 = Select(t=T1."H.Med", s=w263, f=w275) -> (s? t:f=w274:T1)
            n116 = Select(t=T1."H.High", s=w262, f=w274) -> (s? t:f=w273:T1)
            n117 = Select(t=T1."C.Low", s=w261, f=w273) -> (s? t:f=w272:T1)
            n118 = Select(t=T1."C.Med", s=w260, f=w272) -> (s? t:f=w271:T1)
            n119 = Select(t=T1."C.High", s=w259, f=w271) -> (s? t:f=w270:T1)
            n120 = Select(t=T1."Home", s=w258, f=w270) -> (s? t:f=w269:T1)
            n121 = Select(t=T1."Pull Out Grab", s=w257, f=w269) -> (s? t:f=w268:T1)
            n122 = Select(t=T1."Pull Out Release", s=w256, f=w268) -> (s? t:f=w267:T1)
            n123 = Select(t=T1."Pre Climb", s=w255, f=w267) -> (s? t:f=w242:T1)
          }
          frame "H.Low" {
            # "Bag Night Code = 0.5"
            # "Bag Night Code = 0.75"
            # "Bag Night Code = -0.5"
            # "Bag Night Code = -0.75"
            # "Bag Night Code = 18"
            # "Bag Night Code = 18"
            # "Actual Position"
            # "Desired Position"
            # "Below"
            # "Neutral"
            # "Above"
            n124 = Add(x="H Low", y=10) -> (x+y=w298:i32)
            n125 = Subtract(x="H Low", y=10) -> (x-y=w299:i32)
            n126 = In Range and Coerce(upper limit=w298, x=w289, lower limit=w299) -> (In Range?=w294:bool)  [unwired: 1 out]
            n127 = Less?(x="H Low", y=w289) -> (x < y?=w296:bool)
            n128 = Greater?(x="H Low", y=w289) -> (0:w295:bool)
            n129 = case shown="True" w295 {
              tunnel: "H Low" -> [_ w312]
              tunnel: w289 -> [_ w313]
              frame False {
              }
              frame True {
                w320 = T9 0 items=["PercentOutput"=0, "Position"=1, "Velocity"=2, "Current"=3, "Follower"=5, "MotionProfile"=6, "MotionMagic"=7, "MotionProfileArc"=10, "Disabled"=15] ("Control Mode")
                # "50 Org."
                n130 = call <vilib>:"CTRE_Phoenix_MotorControl_RefNumRegistryGet.vi"("refnum name"="Arm Actuator") -> ("PhoenixMotorControlDevRef"=w322:T2)  [unwired: 9 in, 1 out]
                n131 = Subtract(x=w312, y=70) -> (x-y=w316:i32)
                n132 = In Range and Coerce(upper limit=w312, x=w313, lower limit=w316) -> (In Range?=w315:bool)  [unwired: 1 out]
                n133 = Select(t=0.25 ("Output"), s=w315, f=1.0 ("Output")) -> (s? t:f=w314:dbl)
                n134 = call <vilib>:"CTRE_Phoenix_MotorControl_Set.vi"("Output"=w314, "Control Mode"=w320, "PhoenixMotorControlDevRef"=w322) -> ()  [unwired: 7 in, 2 out]
              }
            }
            n135 = case shown="True" w296 {
              tunnel: "H Low" -> [_ w301]
              tunnel: w289 -> [_ w302]
              frame False {
              }
              frame True {
                w309 = T9 0 items=["PercentOutput"=0, "Position"=1, "Velocity"=2, "Current"=3, "Follower"=5, "MotionProfile"=6, "MotionMagic"=7, "MotionProfileArc"=10, "Disabled"=15] ("Control Mode")
                # "50 Org."
                n136 = call <vilib>:"CTRE_Phoenix_MotorControl_RefNumRegistryGet.vi"("refnum name"="Arm Actuator") -> ("PhoenixMotorControlDevRef"=w311:T2)  [unwired: 9 in, 1 out]
                n137 = Add(x=w301, y=70) -> (x+y=w305:i32)
                n138 = In Range and Coerce(upper limit=w305, x=w302, lower limit=w301) -> (In Range?=w303:bool)  [unwired: 1 out]
                n139 = Select(t=-0.25 ("Output"), s=w303, f=-1.0 ("Output")) -> (s? t:f=w308:dbl)
                n140 = call <vilib>:"CTRE_Phoenix_MotorControl_Set.vi"("Output"=w308, "Control Mode"=w309, "PhoenixMotorControlDevRef"=w311) -> ()  [unwired: 7 in, 2 out]
              }
            }
            n141 = Select(t=T1."Wait", s=w294, f=T1."H.Low") -> (s? t:f=w293:T1)
            n142 = call-poly <vilib>:"CTRE_Phoenix_MotorController_Get_Enhanced.vi"("PhoenixMotorControlDevRef"=w291) -> ("AnalogInRaw"=w292:i32)  [unwired: 10 in, 4 out]
          }
          frame "H.Med" {
            # "Actual Position"
            # "Desired Position"
            # "Below"
            # "Neutral"
            # "Above"
            n143 = Add(x="H Med", y=10) -> (x+y=w334:i32)
            n144 = Subtract(x="H Med", y=10) -> (x-y=w335:i32)
            n145 = In Range and Coerce(upper limit=w334, x=w327, lower limit=w335) -> (In Range?=w330:bool)  [unwired: 1 out]
            n146 = Less?(x="H Med", y=w327) -> (x < y?=w332:bool)
            n147 = Greater?(x="H Med", y=w327) -> (0:w331:bool)
            n148 = case shown="True" w332 {
              tunnel: w327 -> [_ w339]
              tunnel: "H Med" -> [_ w338]
              frame False {
              }
              frame True {
                w345 = T9 0 items=["PercentOutput"=0, "Position"=1, "Velocity"=2, "Current"=3, "Follower"=5, "MotionProfile"=6, "MotionMagic"=7, "MotionProfileArc"=10, "Disabled"=15] ("Control Mode")
                n149 = call <vilib>:"CTRE_Phoenix_MotorControl_RefNumRegistryGet.vi"("refnum name"="Arm Actuator") -> ("PhoenixMotorControlDevRef"=w347:T2)  [unwired: 9 in, 1 out]
                n150 = Add(x=w338, y=70) -> (x+y=w342:i32)
                n151 = In Range and Coerce(upper limit=w342, x=w339, lower limit=w338) -> (In Range?=w340:bool)  [unwired: 1 out]
                n152 = Select(t=-0.25 ("Output"), s=w340, f=-1.0 ("Output")) -> (s? t:f=w337:dbl)
                n153 = call <vilib>:"CTRE_Phoenix_MotorControl_Set.vi"("Output"=w337, "Control Mode"=w345, "PhoenixMotorControlDevRef"=w347) -> ()  [unwired: 7 in, 2 out]
              }
            }
            n154 = case shown="True" w331 {
              tunnel: "H Med" -> [_ w349]
              tunnel: w327 -> [_ w348]
              frame False {
              }
              frame True {
                w356 = T9 0 items=["PercentOutput"=0, "Position"=1, "Velocity"=2, "Current"=3, "Follower"=5, "MotionProfile"=6, "MotionMagic"=7, "MotionProfileArc"=10, "Disabled"=15] ("Control Mode")
                n155 = call <vilib>:"CTRE_Phoenix_MotorControl_RefNumRegistryGet.vi"("refnum name"="Arm Actuator") -> ("PhoenixMotorControlDevRef"=w358:T2)  [unwired: 9 in, 1 out]
                n156 = Subtract(x=w349, y=70) -> (x-y=w352:i32)
                n157 = In Range and Coerce(upper limit=w349, x=w348, lower limit=w352) -> (In Range?=w351:bool)  [unwired: 1 out]
                n158 = Select(t=0.25 ("Output"), s=w351, f=1.0 ("Output")) -> (s? t:f=w350:dbl)
                n159 = call <vilib>:"CTRE_Phoenix_MotorControl_Set.vi"("Output"=w350, "Control Mode"=w356, "PhoenixMotorControlDevRef"=w358) -> ()  [unwired: 7 in, 2 out]
              }
            }
            n160 = Select(t=T1."Wait", s=w330, f=T1."H.Med") -> (s? t:f=w329:T1)
            n161 = call-poly <vilib>:"CTRE_Phoenix_MotorController_Get_Enhanced.vi"("PhoenixMotorControlDevRef"=w325) -> ("AnalogInRaw"=w328:i32)  [unwired: 10 in, 4 out]
          }
          frame "H.High" {
            # "Actual Position"
            # "Desired Position"
            # "Below"
            # "Neutral"
            # "Above"
            n162 = Add(x="H High", y=10) -> (x+y=w370:i32)
            n163 = Subtract(x="H High", y=10) -> (x-y=w371:i32)
            n164 = In Range and Coerce(upper limit=w370, x=w362, lower limit=w371) -> (In Range?=w367:bool)  [unwired: 1 out]
            n165 = Less?(x="H High", y=w362) -> (x < y?=w365:bool)
            n166 = Greater?(x="H High", y=w362) -> (0:w368:bool)
            n167 = case shown="True" w368 {
              tunnel: w362 -> [_ w385]
              tunnel: "H High" -> [_ w384]
              frame False {
              }
              frame True {
                w392 = T9 0 items=["PercentOutput"=0, "Position"=1, "Velocity"=2, "Current"=3, "Follower"=5, "MotionProfile"=6, "MotionMagic"=7, "MotionProfileArc"=10, "Disabled"=15] ("Control Mode")
                n168 = call <vilib>:"CTRE_Phoenix_MotorControl_RefNumRegistryGet.vi"("refnum name"="Arm Actuator") -> ("PhoenixMotorControlDevRef"=w394:T2)  [unwired: 9 in, 1 out]
                n169 = Subtract(x=w384, y=70) -> (x-y=w388:i32)
                n170 = In Range and Coerce(upper limit=w384, x=w385, lower limit=w388) -> (In Range?=w387:bool)  [unwired: 1 out]
                n171 = Select(t=0.25 ("Output"), s=w387, f=1.0 ("Output")) -> (s? t:f=w386:dbl)
                n172 = call <vilib>:"CTRE_Phoenix_MotorControl_Set.vi"("Output"=w386, "Control Mode"=w392, "PhoenixMotorControlDevRef"=w394) -> ()  [unwired: 7 in, 2 out]
              }
            }
            n173 = case shown="True" w365 {
              tunnel: w362 -> [_ w374]
              tunnel: "H High" -> [_ w373]
              frame False {
              }
              frame True {
                w381 = T9 0 items=["PercentOutput"=0, "Position"=1, "Velocity"=2, "Current"=3, "Follower"=5, "MotionProfile"=6, "MotionMagic"=7, "MotionProfileArc"=10, "Disabled"=15] ("Control Mode")
                n174 = call <vilib>:"CTRE_Phoenix_MotorControl_RefNumRegistryGet.vi"("refnum name"="Arm Actuator") -> ("PhoenixMotorControlDevRef"=w383:T2)  [unwired: 9 in, 1 out]
                n175 = Add(x=w373, y=70) -> (x+y=w378:i32)
                n176 = In Range and Coerce(upper limit=w378, x=w374, lower limit=w373) -> (In Range?=w376:bool)  [unwired: 1 out]
                n177 = Select(t=-0.25 ("Output"), s=w376, f=-1.0 ("Output")) -> (s? t:f=w375:dbl)
                n178 = call <vilib>:"CTRE_Phoenix_MotorControl_Set.vi"("Output"=w375, "Control Mode"=w381, "PhoenixMotorControlDevRef"=w383) -> ()  [unwired: 7 in, 2 out]
              }
            }
            n179 = Select(t=T1."Wait", s=w367, f=T1."H.High") -> (s? t:f=w366:T1)
            n180 = call-poly <vilib>:"CTRE_Phoenix_MotorController_Get_Enhanced.vi"("PhoenixMotorControlDevRef"=w363) -> ("AnalogInRaw"=w364:i32)  [unwired: 10 in, 4 out]
          }
          frame "C.Low" {
            # "Actual Position"
            # "Desired Position"
            # "Below"
            # "Neutral"
            # "Above"
            n181 = Add(x="C Low", y=10) -> (x+y=w406:i32)
            n182 = Subtract(x="C Low", y=10) -> (x-y=w407:i32)
            n183 = In Range and Coerce(upper limit=w406, x=w398, lower limit=w407) -> (In Range?=w403:bool)  [unwired: 1 out]
            n184 = Less?(x="C Low", y=w398) -> (x < y?=w402:bool)
            n185 = Greater?(x="C Low", y=w398) -> (0:w404:bool)
            n186 = case shown="True" w404 {
              tunnel: w398 -> [_ w421]
              tunnel: "C Low" -> [_ w420]
              frame False {
              }
              frame True {
                w428 = T9 0 items=["PercentOutput"=0, "Position"=1, "Velocity"=2, "Current"=3, "Follower"=5, "MotionProfile"=6, "MotionMagic"=7, "MotionProfileArc"=10, "Disabled"=15] ("Control Mode")
                n187 = call <vilib>:"CTRE_Phoenix_MotorControl_RefNumRegistryGet.vi"("refnum name"="Arm Actuator") -> ("PhoenixMotorControlDevRef"=w430:T2)  [unwired: 9 in, 1 out]
                n188 = Subtract(x=w420, y=70) -> (x-y=w424:i32)
                n189 = In Range and Coerce(upper limit=w420, x=w421, lower limit=w424) -> (In Range?=w423:bool)  [unwired: 1 out]
                n190 = Select(t=0.25 ("Output"), s=w423, f=1.0 ("Output")) -> (s? t:f=w422:dbl)
                n191 = call <vilib>:"CTRE_Phoenix_MotorControl_Set.vi"("Output"=w422, "Control Mode"=w428, "PhoenixMotorControlDevRef"=w430) -> ()  [unwired: 7 in, 2 out]
              }
            }
            n192 = case shown="True" w402 {
              tunnel: w398 -> [_ w410]
              tunnel: "C Low" -> [_ w409]
              frame False {
              }
              frame True {
                w417 = T9 0 items=["PercentOutput"=0, "Position"=1, "Velocity"=2, "Current"=3, "Follower"=5, "MotionProfile"=6, "MotionMagic"=7, "MotionProfileArc"=10, "Disabled"=15] ("Control Mode")
                n193 = call <vilib>:"CTRE_Phoenix_MotorControl_RefNumRegistryGet.vi"("refnum name"="Arm Actuator") -> ("PhoenixMotorControlDevRef"=w419:T2)  [unwired: 9 in, 1 out]
                n194 = Add(x=w409, y=70) -> (x+y=w414:i32)
                n195 = In Range and Coerce(upper limit=w414, x=w410, lower limit=w409) -> (In Range?=w412:bool)  [unwired: 1 out]
                n196 = Select(t=-0.25 ("Output"), s=w412, f=-1.0 ("Output")) -> (s? t:f=w411:dbl)
                n197 = call <vilib>:"CTRE_Phoenix_MotorControl_Set.vi"("Output"=w411, "Control Mode"=w417, "PhoenixMotorControlDevRef"=w419) -> ()  [unwired: 7 in, 2 out]
              }
            }
            n198 = Select(t=T1."Wait", s=w403, f=T1."C.Low") -> (s? t:f=w401:T1)
            n199 = call-poly <vilib>:"CTRE_Phoenix_MotorController_Get_Enhanced.vi"("PhoenixMotorControlDevRef"=w399) -> ("AnalogInRaw"=w400:i32)  [unwired: 10 in, 4 out]
          }
          frame "C.Med" {
            # "Actual Position"
            # "Desired Position"
            # "Below"
            # "Neutral"
            # "Above"
            n200 = Add(x="C Med", y=10) -> (x+y=w442:i32)
            n201 = Subtract(x="C Med", y=10) -> (x-y=w443:i32)
            n202 = In Range and Coerce(upper limit=w442, x=w434, lower limit=w443) -> (In Range?=w439:bool)  [unwired: 1 out]
            n203 = Less?(x="C Med", y=w434) -> (x < y?=w438:bool)
            n204 = Greater?(x="C Med", y=w434) -> (0:w440:bool)
            n205 = case shown="True" w440 {
              tunnel: w434 -> [_ w457]
              tunnel: "C Med" -> [_ w456]
              frame False {
              }
              frame True {
                w464 = T9 0 items=["PercentOutput"=0, "Position"=1, "Velocity"=2, "Current"=3, "Follower"=5, "MotionProfile"=6, "MotionMagic"=7, "MotionProfileArc"=10, "Disabled"=15] ("Control Mode")
                n206 = call <vilib>:"CTRE_Phoenix_MotorControl_RefNumRegistryGet.vi"("refnum name"="Arm Actuator") -> ("PhoenixMotorControlDevRef"=w466:T2)  [unwired: 9 in, 1 out]
                n207 = Subtract(x=w456, y=70) -> (x-y=w460:i32)
                n208 = In Range and Coerce(upper limit=w456, x=w457, lower limit=w460) -> (In Range?=w459:bool)  [unwired: 1 out]
                n209 = Select(t=0.25 ("Output"), s=w459, f=1.0 ("Output")) -> (s? t:f=w458:dbl)
                n210 = call <vilib>:"CTRE_Phoenix_MotorControl_Set.vi"("Output"=w458, "Control Mode"=w464, "PhoenixMotorControlDevRef"=w466) -> ()  [unwired: 7 in, 2 out]
              }
            }
            n211 = case shown="True" w438 {
              tunnel: w434 -> [_ w446]
              tunnel: "C Med" -> [_ w445]
              frame False {
              }
              frame True {
                w453 = T9 0 items=["PercentOutput"=0, "Position"=1, "Velocity"=2, "Current"=3, "Follower"=5, "MotionProfile"=6, "MotionMagic"=7, "MotionProfileArc"=10, "Disabled"=15] ("Control Mode")
                n212 = call <vilib>:"CTRE_Phoenix_MotorControl_RefNumRegistryGet.vi"("refnum name"="Arm Actuator") -> ("PhoenixMotorControlDevRef"=w455:T2)  [unwired: 9 in, 1 out]
                n213 = Add(x=w445, y=70) -> (x+y=w450:i32)
                n214 = In Range and Coerce(upper limit=w450, x=w446, lower limit=w445) -> (In Range?=w448:bool)  [unwired: 1 out]
                n215 = Select(t=-0.25 ("Output"), s=w448, f=-1.0 ("Output")) -> (s? t:f=w447:dbl)
                n216 = call <vilib>:"CTRE_Phoenix_MotorControl_Set.vi"("Output"=w447, "Control Mode"=w453, "PhoenixMotorControlDevRef"=w455) -> ()  [unwired: 7 in, 2 out]
              }
            }
            n217 = Select(t=T1."Wait", s=w439, f=T1."C.Med") -> (s? t:f=w437:T1)
            n218 = call-poly <vilib>:"CTRE_Phoenix_MotorController_Get_Enhanced.vi"("PhoenixMotorControlDevRef"=w435) -> ("AnalogInRaw"=w436:i32)  [unwired: 10 in, 4 out]
          }
          frame "C.High" {
            # "Actual Position"
            # "Desired Position"
            # "Below"
            # "Neutral"
            # "Above"
            n219 = Add(x="C High", y=10) -> (x+y=w478:i32)
            n220 = Subtract(x="C High", y=10) -> (x-y=w479:i32)
            n221 = In Range and Coerce(upper limit=w478, x=w470, lower limit=w479) -> (In Range?=w476:bool)  [unwired: 1 out]
            n222 = Less?(x="C High", y=w470) -> (x < y?=w473:bool)
            n223 = Greater?(x="C High", y=w470) -> (0:w474:bool)
            n224 = case shown="True" w473 {
              tunnel: w470 -> [_ w482]
              tunnel: "C High" -> [_ w481]
              frame False {
              }
              frame True {
                w489 = T9 0 items=["PercentOutput"=0, "Position"=1, "Velocity"=2, "Current"=3, "Follower"=5, "MotionProfile"=6, "MotionMagic"=7, "MotionProfileArc"=10, "Disabled"=15] ("Control Mode")
                n225 = call <vilib>:"CTRE_Phoenix_MotorControl_RefNumRegistryGet.vi"("refnum name"="Arm Actuator") -> ("PhoenixMotorControlDevRef"=w491:T2)  [unwired: 9 in, 1 out]
                n226 = Add(x=w481, y=70) -> (x+y=w486:i32)
                n227 = In Range and Coerce(upper limit=w486, x=w482, lower limit=w481) -> (In Range?=w484:bool)  [unwired: 1 out]
                n228 = Select(t=-0.25 ("Output"), s=w484, f=-1.0 ("Output")) -> (s? t:f=w483:dbl)
                n229 = call <vilib>:"CTRE_Phoenix_MotorControl_Set.vi"("Output"=w483, "Control Mode"=w489, "PhoenixMotorControlDevRef"=w491) -> ()  [unwired: 7 in, 2 out]
              }
            }
            n230 = case shown="True" w474 {
              tunnel: w470 -> [_ w493]
              tunnel: "C High" -> [_ w492]
              frame False {
              }
              frame True {
                w500 = T9 0 items=["PercentOutput"=0, "Position"=1, "Velocity"=2, "Current"=3, "Follower"=5, "MotionProfile"=6, "MotionMagic"=7, "MotionProfileArc"=10, "Disabled"=15] ("Control Mode")
                n231 = call <vilib>:"CTRE_Phoenix_MotorControl_RefNumRegistryGet.vi"("refnum name"="Arm Actuator") -> ("PhoenixMotorControlDevRef"=w502:T2)  [unwired: 9 in, 1 out]
                n232 = Subtract(x=w493, y=70) -> (x-y=w496:i32)
                n233 = In Range and Coerce(upper limit=w493, x=w492, lower limit=w496) -> (In Range?=w495:bool)  [unwired: 1 out]
                n234 = Select(t=0.25 ("Output"), s=w495, f=1.0 ("Output")) -> (s? t:f=w494:dbl)
                n235 = call <vilib>:"CTRE_Phoenix_MotorControl_Set.vi"("Output"=w494, "Control Mode"=w500, "PhoenixMotorControlDevRef"=w502) -> ()  [unwired: 7 in, 2 out]
              }
            }
            n236 = Select(t=T1."Wait", s=w476, f=T1."C.High") -> (s? t:f=w475:T1)
            n237 = call-poly <vilib>:"CTRE_Phoenix_MotorController_Get_Enhanced.vi"("PhoenixMotorControlDevRef"=w471) -> ("AnalogInRaw"=w472:i32)  [unwired: 10 in, 4 out]
          }
          frame "Home" {
            # "Bag Night Code = 0.4"
            # "Bag Night Code = -0.75"
            # "Bag Night Code = 0.4"
            # "Bag Night Code = 0.75"
            # "Actual Position"
            # "Desired Position"
            # "Below"
            # "Neutral"
            # "Above"
            n238 = Add(x="Home", y=18) -> (x+y=w514:i32)
            n239 = Subtract(x="Home", y=18) -> (x-y=w515:i32)
            n240 = In Range and Coerce(upper limit=w514, x=w506, lower limit=w515) -> (In Range?=w512:bool)  [unwired: 1 out]
            n241 = Less?(x="Home", y=w506) -> (x < y?=w510:bool)
            n242 = Greater?(x="Home", y=w506) -> (0:w511:bool)
            n243 = case shown="True" w511 {
              tunnel: w506 -> [_ w530]
              tunnel: "Home" -> [_ w529]
              frame False {
              }
              frame True {
                w536 = T9 0 items=["PercentOutput"=0, "Position"=1, "Velocity"=2, "Current"=3, "Follower"=5, "MotionProfile"=6, "MotionMagic"=7, "MotionProfileArc"=10, "Disabled"=15] ("Control Mode")
                n244 = call <vilib>:"CTRE_Phoenix_MotorControl_RefNumRegistryGet.vi"("refnum name"="Arm Actuator") -> ("PhoenixMotorControlDevRef"=w538:T2)  [unwired: 9 in, 1 out]
                n245 = Subtract(x=w529, y=50) -> (x-y=w532:i32)
                n246 = In Range and Coerce(upper limit=w529, x=w530, lower limit=w532) -> (In Range?=w531:bool)  [unwired: 1 out]
                n247 = Select(t=0.25 ("Output"), s=w531, f=0.5 ("Output")) -> (s? t:f=w528:dbl)
                n248 = call <vilib>:"CTRE_Phoenix_MotorControl_Set.vi"("Output"=w528, "Control Mode"=w536, "PhoenixMotorControlDevRef"=w538) -> ()  [unwired: 7 in, 2 out]
              }
            }
            n249 = case shown="True" w510 {
              tunnel: w506 -> [_ w518]
              tunnel: "Home" -> [_ w517]
              frame False {
              }
              frame True {
                w525 = T9 0 items=["PercentOutput"=0, "Position"=1, "Velocity"=2, "Current"=3, "Follower"=5, "MotionProfile"=6, "MotionMagic"=7, "MotionProfileArc"=10, "Disabled"=15] ("Control Mode")
                n250 = call <vilib>:"CTRE_Phoenix_MotorControl_RefNumRegistryGet.vi"("refnum name"="Arm Actuator") -> ("PhoenixMotorControlDevRef"=w527:T2)  [unwired: 9 in, 1 out]
                n251 = Add(x=w517, y=50) -> (x+y=w522:i32)
                n252 = In Range and Coerce(upper limit=w522, x=w518, lower limit=w517) -> (In Range?=w520:bool)  [unwired: 1 out]
                n253 = Select(t=-0.25 ("Output"), s=w520, f=-0.5 ("Output")) -> (s? t:f=w519:dbl)
                n254 = call <vilib>:"CTRE_Phoenix_MotorControl_Set.vi"("Output"=w519, "Control Mode"=w525, "PhoenixMotorControlDevRef"=w527) -> ()  [unwired: 7 in, 2 out]
              }
            }
            n255 = Select(t=T1."Wait", s=w512, f=T1."Home") -> (s? t:f=w509:T1)
            n256 = call-poly <vilib>:"CTRE_Phoenix_MotorController_Get_Enhanced.vi"("PhoenixMotorControlDevRef"=w507) -> ("AnalogInRaw"=w508:i32)  [unwired: 10 in, 4 out]
          }
          frame "Pull Out Grab" {
            # "Uses a sequence structure to move the claw up and backwards to pick up hatches"
            n257 = case shown="True" w544 {
              tunnel: w539 -> [_ w548]
              tunnel: w543 -> [w545 _]
              tunnel: [w545 w546] -> w542
              tunnel: w541 -> [_ w547]
              frame False {
              }
              frame True {
                n258 = flat-sequence {
                  tunnel: w548 -> [w550]
                  tunnel: w547 -> [w557]
                  tunnel: [T1."Wait"] -> w546
                  frame #0 {
                    # "Claw Up\nHigh enough to take the hatch."
                    n259 = for {
                      N: "Grab Time" -> [_]
                      tunnel: w550 -> [w554]
                      w553 = T9 0 items=["PercentOutput"=0, "Position"=1, "Velocity"=2, "Current"=3, "Follower"=5, "MotionProfile"=6, "MotionMagic"=7, "MotionProfileArc"=10, "Disabled"=15] ("Control Mode")
                      n260 = call <vilib>:"CTRE_Phoenix_MotorControl_Set.vi"("Output"=0.65, "Control Mode"=w553, "PhoenixMotorControlDevRef"=w554) -> ()  [unwired: 7 in, 2 out]
                      n261 = Wait (ms)(milliseconds to wait=u32 25) -> ()  [unwired: 1 out]
                    }
                  }
                  frame #1 {
                    n262 = for {
                      N: "Grab Wait Time" -> [_]
                      n263 = Wait (ms)(milliseconds to wait=u32 25) -> ()  [unwired: 1 out]
                    }
                  }
                  frame #2 {
                    # "Back Up\nFar enough to not interfere with the field."
                    n264 = for {
                      N: "Grab Drive Time" -> [_]
                      tunnel: w557 -> [w561]
                      # "Keep x, and rotation axies 0"
                      n265 = call-poly <vilib>:"WPI_RobotDriveHolonomicDrive.vi"("Rotation"=0.0, "Y"=0.5, "X"=0.0, "RobotDriveDevRef"=w561) -> ()  [unwired: 5 in, 3 out]
                      n266 = Wait (ms)(milliseconds to wait=u32 25) -> ()  [unwired: 1 out]
                    }
                  }
                  frame #3 {
                  }
                }
              }
            }
            n267 = call-poly <vilib>:"CTRE_Phoenix_MotorController_Get_Enhanced.vi"("PhoenixMotorControlDevRef"=w539) -> ("AnalogInRaw"=w540:i32)  [unwired: 10 in, 4 out]
          }
          frame "Pull Out Release" {
            # "Uses a sequence structure to move the claw down and backwards inorder to place the hatches"
            n268 = case shown="True" w569 {
              tunnel: w565 -> [_ w574]
              tunnel: w570 -> [w571 _]
              tunnel: [w571 w573] -> w568
              tunnel: w567 -> [_ w572]
              frame False {
              }
              frame True {
                n269 = flat-sequence {
                  tunnel: w574 -> [w577]
                  tunnel: w572 -> [w575]
                  tunnel: [T1."Wait"] -> w573
                  frame #0 {
                    # "Arm Down\nFar enough to let go of the hatch panel."
                    n270 = for {
                      N: "Release Time" -> [_]
                      tunnel: w577 -> [w585]
                      tunnel: w575 -> [w578]
                      w584 = T9 0 items=["PercentOutput"=0, "Position"=1, "Velocity"=2, "Current"=3, "Follower"=5, "MotionProfile"=6, "MotionMagic"=7, "MotionProfileArc"=10, "Disabled"=15] ("Control Mode")
                      # "Keep x, and rotation axies 0"
                      n271 = call-poly <vilib>:"WPI_RobotDriveHolonomicDrive.vi"("Rotation"=0.0, "Y"=0.5, "X"=0.0, "RobotDriveDevRef"=w578) -> ()  [unwired: 5 in, 3 out]
                      n272 = call <vilib>:"CTRE_Phoenix_MotorControl_Set.vi"("Output"=-0.55, "Control Mode"=w584, "PhoenixMotorControlDevRef"=w585) -> ()  [unwired: 7 in, 2 out]
                      n273 = Wait (ms)(milliseconds to wait=u32 25) -> ()  [unwired: 1 out]
                    }
                  }
                  frame #1 {
                  }
                }
              }
            }
            n274 = call-poly <vilib>:"CTRE_Phoenix_MotorController_Get_Enhanced.vi"("PhoenixMotorControlDevRef"=w565) -> ("AnalogInRaw"=w566:i32)  [unwired: 10 in, 4 out]
          }
          frame "Pre Climb" {
            # "Actual Position"
            # "Desired Position"
            # "Below"
            # "Neutral"
            # "Above"
            n275 = Add(x="Pre Climb", y=20) -> (x+y=w598:i32)
            n276 = Subtract(x="Pre Climb", y=20) -> (x-y=w599:i32)
            n277 = In Range and Coerce(upper limit=w598, x=w591, lower limit=w599) -> (In Range?=w594:bool)  [unwired: 1 out]
            n278 = Less?(x="Pre Climb", y=w591) -> (x < y?=w596:bool)
            n279 = Greater?(x="Pre Climb", y=w591) -> (0:w595:bool)
            n280 = case shown="True" w595 {
              tunnel: "Pre Climb" -> [_ w612]
              tunnel: w591 -> [_ w613]
              frame False {
              }
              frame True {
                w620 = T9 0 items=["PercentOutput"=0, "Position"=1, "Velocity"=2, "Current"=3, "Follower"=5, "MotionProfile"=6, "MotionMagic"=7, "MotionProfileArc"=10, "Disabled"=15] ("Control Mode")
                n281 = call <vilib>:"CTRE_Phoenix_MotorControl_RefNumRegistryGet.vi"("refnum name"="Arm Actuator") -> ("PhoenixMotorControlDevRef"=w622:T2)  [unwired: 9 in, 1 out]
                n282 = Subtract(x=w612, y=50) -> (x-y=w616:i32)
                n283 = In Range and Coerce(upper limit=w612, x=w613, lower limit=w616) -> (In Range?=w615:bool)  [unwired: 1 out]
                n284 = Select(t=0.25 ("Output"), s=w615, f=0.5 ("Output")) -> (s? t:f=w614:dbl)
                n285 = call <vilib>:"CTRE_Phoenix_MotorControl_Set.vi"("Output"=w614, "Control Mode"=w620, "PhoenixMotorControlDevRef"=w622) -> ()  [unwired: 7 in, 2 out]
              }
            }
            n286 = case shown="True" w596 {
              tunnel: "Pre Climb" -> [_ w601]
              tunnel: w591 -> [_ w602]
              frame False {
              }
              frame True {
                w609 = T9 0 items=["PercentOutput"=0, "Position"=1, "Velocity"=2, "Current"=3, "Follower"=5, "MotionProfile"=6, "MotionMagic"=7, "MotionProfileArc"=10, "Disabled"=15] ("Control Mode")
                n287 = call <vilib>:"CTRE_Phoenix_MotorControl_RefNumRegistryGet.vi"("refnum name"="Arm Actuator") -> ("PhoenixMotorControlDevRef"=w611:T2)  [unwired: 9 in, 1 out]
                n288 = Add(x=w601, y=50) -> (x+y=w605:i32)
                n289 = In Range and Coerce(upper limit=w605, x=w602, lower limit=w601) -> (In Range?=w603:bool)  [unwired: 1 out]
                n290 = Select(t=-0.25 ("Output"), s=w603, f=-0.5 ("Output")) -> (s? t:f=w608:dbl)
                n291 = call <vilib>:"CTRE_Phoenix_MotorControl_Set.vi"("Output"=w608, "Control Mode"=w609, "PhoenixMotorControlDevRef"=w611) -> ()  [unwired: 7 in, 2 out]
              }
            }
            n292 = Select(t=T1."Upward Travel", s=w594, f=T1."Pre Climb") -> (s? t:f=w590:T1)
            n293 = call-poly <vilib>:"CTRE_Phoenix_MotorController_Get_Enhanced.vi"("PhoenixMotorControlDevRef"=w592) -> ("AnalogInRaw"=w589:i32)  [unwired: 10 in, 4 out]
          }
          frame "Upward Travel" {
            # "Jack Foot"
            # "Jack"
            # "Arm"
            # "Uses the arm and jack to climb the habitat's side"
            n294 = for {
              N: 116 -> [_]
              tunnel: w631 -> [w645]
              tunnel: "Arm speed" -> [w644]
              tunnel: "Jack speed 1" -> [w643]
              tunnel: w628 -> [w642]
              tunnel: w627 -> [w638]
              tunnel: [w635] -> w624
              w639 = T9 0 items=["PercentOutput"=0, "Position"=1, "Velocity"=2, "Current"=3, "Follower"=5, "MotionProfile"=6, "MotionMagic"=7, "MotionProfileArc"=10, "Disabled"=15] ("Control Mode")
              w640 = T9 0 items=["PercentOutput"=0, "Position"=1, "Velocity"=2, "Current"=3, "Follower"=5, "MotionProfile"=6, "MotionMagic"=7, "MotionProfileArc"=10, "Disabled"=15] ("Control Mode")
              w641 = T9 0 items=["PercentOutput"=0, "Position"=1, "Velocity"=2, "Current"=3, "Follower"=5, "MotionProfile"=6, "MotionMagic"=7, "MotionProfileArc"=10, "Disabled"=15] ("Control Mode")
              n295 = call <vilib>:"CTRE_Phoenix_MotorControl_Set.vi"("Output"=w644, "Control Mode"=w640, "PhoenixMotorControlDevRef"=w645) -> ()  [unwired: 7 in, 2 out]
              n296 = call <vilib>:"CTRE_Phoenix_MotorControl_Set.vi"("Output"=w643, "Control Mode"=w641, "PhoenixMotorControlDevRef"=w642) -> ()  [unwired: 7 in, 2 out]
              n297 = call <vilib>:"CTRE_Phoenix_MotorControl_Set.vi"("Output"=0.0, "Control Mode"=w639, "PhoenixMotorControlDevRef"=w638) -> ("PhoenixMotorControlDevRef"=w635:T2)  [unwired: 7 in, 1 out]
              n298 = Wait (ms)(milliseconds to wait=u32 10) -> ()  [unwired: 1 out]
            }
            n299 = for {
              N: 1 -> [_]
              tunnel: [T1."Extra Jack Time"] -> w625
              tunnel: w624 -> [_]
              n300 = Wait (ms)(milliseconds to wait=u32 10) -> ()  [unwired: 1 out]
            }
          }
          frame "Extra Jack Time" {
            # "extra time given to jack the back end up to get more clearance on the platform"
            # "Jack Foot"
            # "Jack"
            # "Arm"
            n301 = for {
              N: 217 -> [_]
              tunnel: w653 -> [w667]
              tunnel: w652 -> [w666]
              tunnel: w651 -> [w665]
              tunnel: "Jack speed 2" -> [w661]
              tunnel: [w657] -> w648
              w662 = T9 0 items=["PercentOutput"=0, "Position"=1, "Velocity"=2, "Current"=3, "Follower"=5, "MotionProfile"=6, "MotionMagic"=7, "MotionProfileArc"=10, "Disabled"=15] ("Control Mode")
              w663 = T9 0 items=["PercentOutput"=0, "Position"=1, "Velocity"=2, "Current"=3, "Follower"=5, "MotionProfile"=6, "MotionMagic"=7, "MotionProfileArc"=10, "Disabled"=15] ("Control Mode")
              w664 = T9 0 items=["PercentOutput"=0, "Position"=1, "Velocity"=2, "Current"=3, "Follower"=5, "MotionProfile"=6, "MotionMagic"=7, "MotionProfileArc"=10, "Disabled"=15] ("Control Mode")
              n302 = call <vilib>:"CTRE_Phoenix_MotorControl_Set.vi"("Output"=0.0, "Control Mode"=w664, "PhoenixMotorControlDevRef"=w667) -> ()  [unwired: 7 in, 2 out]
              n303 = call <vilib>:"CTRE_Phoenix_MotorControl_Set.vi"("Output"=w661, "Control Mode"=w663, "PhoenixMotorControlDevRef"=w666) -> ()  [unwired: 7 in, 2 out]
              n304 = call <vilib>:"CTRE_Phoenix_MotorControl_Set.vi"("Output"=0.0, "Control Mode"=w662, "PhoenixMotorControlDevRef"=w665) -> ("PhoenixMotorControlDevRef"=w657:T2)  [unwired: 7 in, 1 out]
              n305 = Wait (ms)(milliseconds to wait=u32 10) -> ()  [unwired: 1 out]
            }
            n306 = for {
              N: 1 -> [_]
              tunnel: w648 -> [_]
              tunnel: [T1."Forward Travel"] -> w647
              n307 = Wait (ms)(milliseconds to wait=u32 10) -> ()  [unwired: 1 out]
            }
          }
          frame "Forward Travel" {
            # "Bring the robot forward onto the platform by running the jack foot"
            # "Jack Foot"
            # "Jack"
            # "Arm"
            n308 = for {
              N: 230 -> [_]
              tunnel: w675 -> [w689]
              tunnel: w674 -> [w688]
              tunnel: w673 -> [w687]
              tunnel: "Jack drive 1" -> [w683]
              tunnel: [w679] -> w668
              w684 = T9 0 items=["PercentOutput"=0, "Position"=1, "Velocity"=2, "Current"=3, "Follower"=5, "MotionProfile"=6, "MotionMagic"=7, "MotionProfileArc"=10, "Disabled"=15] ("Control Mode")
              w685 = T9 0 items=["PercentOutput"=0, "Position"=1, "Velocity"=2, "Current"=3, "Follower"=5, "MotionProfile"=6, "MotionMagic"=7, "MotionProfileArc"=10, "Disabled"=15] ("Control Mode")
              w686 = T9 0 items=["PercentOutput"=0, "Position"=1, "Velocity"=2, "Current"=3, "Follower"=5, "MotionProfile"=6, "MotionMagic"=7, "MotionProfileArc"=10, "Disabled"=15] ("Control Mode")
              n309 = Wait (ms)(milliseconds to wait=u32 10) -> ()  [unwired: 1 out]
              n310 = call <vilib>:"CTRE_Phoenix_MotorControl_Set.vi"("Output"=0.0, "Control Mode"=w685, "PhoenixMotorControlDevRef"=w689) -> ()  [unwired: 7 in, 2 out]
              n311 = call <vilib>:"CTRE_Phoenix_MotorControl_Set.vi"("Output"=0.0, "Control Mode"=w686, "PhoenixMotorControlDevRef"=w688) -> ()  [unwired: 7 in, 2 out]
              n312 = call <vilib>:"CTRE_Phoenix_MotorControl_Set.vi"("Output"=w683, "Control Mode"=w684, "PhoenixMotorControlDevRef"=w687) -> ("PhoenixMotorControlDevRef"=w679:T2)  [unwired: 7 in, 1 out]
            }
            n313 = for {
              N: 1 -> [_]
              tunnel: [T1."Jack Retrieval"] -> w670
              tunnel: w668 -> [_]
              n314 = Wait (ms)(milliseconds to wait=u32 10) -> ()  [unwired: 1 out]
            }
          }
          frame "Jack Retrieval" {
            # "bring the jack back up into the robot so we can be completely supported by the hab platform"
            # "Jack Foot"
            # "Jack"
            # "Arm"
            n315 = for {
              N: 325 -> [_]
              tunnel: w697 -> [w711]
              tunnel: w696 -> [w710]
              tunnel: w695 -> [w709]
              tunnel: "Jack speed 3" -> [w705]
              tunnel: [w701] -> w690
              w706 = T9 0 items=["PercentOutput"=0, "Position"=1, "Velocity"=2, "Current"=3, "Follower"=5, "MotionProfile"=6, "MotionMagic"=7, "MotionProfileArc"=10, "Disabled"=15] ("Control Mode")
              w707 = T9 0 items=["PercentOutput"=0, "Position"=1, "Velocity"=2, "Current"=3, "Follower"=5, "MotionProfile"=6, "MotionMagic"=7, "MotionProfileArc"=10, "Disabled"=15] ("Control Mode")
              w708 = T9 0 items=["PercentOutput"=0, "Position"=1, "Velocity"=2, "Current"=3, "Follower"=5, "MotionProfile"=6, "MotionMagic"=7, "MotionProfileArc"=10, "Disabled"=15] ("Control Mode")
              n316 = Wait (ms)(milliseconds to wait=u32 10) -> ()  [unwired: 1 out]
              n317 = call <vilib>:"CTRE_Phoenix_MotorControl_Set.vi"("Output"=0.0, "Control Mode"=w708, "PhoenixMotorControlDevRef"=w711) -> ()  [unwired: 7 in, 2 out]
              n318 = call <vilib>:"CTRE_Phoenix_MotorControl_Set.vi"("Output"=w705, "Control Mode"=w707, "PhoenixMotorControlDevRef"=w710) -> ()  [unwired: 7 in, 2 out]
              n319 = call <vilib>:"CTRE_Phoenix_MotorControl_Set.vi"("Output"=0.0, "Control Mode"=w706, "PhoenixMotorControlDevRef"=w709) -> ("PhoenixMotorControlDevRef"=w701:T2)  [unwired: 7 in, 1 out]
            }
            n320 = for {
              N: 1 -> [_]
              tunnel: [T1."Wait"] -> w692
              tunnel: w690 -> [_]
              n321 = Wait (ms)(milliseconds to wait=u32 10) -> ()  [unwired: 1 out]
            }
          }
          frame "Load Cargo" {
            # "Actual Position"
            # "Desired Position"
            # "Below"
            # "Neutral"
            # "Above"
            n322 = Add(x="Load Cargo", y=10) -> (x+y=w723:i32)
            n323 = Subtract(x="Load Cargo", y=10) -> (x-y=w724:i32)
            n324 = In Range and Coerce(upper limit=w723, x=w716, lower limit=w724) -> (In Range?=w719:bool)  [unwired: 1 out]
            n325 = Less?(x="Load Cargo", y=w716) -> (x < y?=w721:bool)
            n326 = Greater?(x="Load Cargo", y=w716) -> (0:w720:bool)
            n327 = case shown="True" w720 {
              tunnel: "Load Cargo" -> [_ w737]
              tunnel: w716 -> [_ w738]
              frame False {
              }
              frame True {
                w745 = T9 0 items=["PercentOutput"=0, "Position"=1, "Velocity"=2, "Current"=3, "Follower"=5, "MotionProfile"=6, "MotionMagic"=7, "MotionProfileArc"=10, "Disabled"=15] ("Control Mode")
                n328 = call <vilib>:"CTRE_Phoenix_MotorControl_RefNumRegistryGet.vi"("refnum name"="Arm Actuator") -> ("PhoenixMotorControlDevRef"=w747:T2)  [unwired: 9 in, 1 out]
                n329 = Subtract(x=w737, y=70) -> (x-y=w741:i32)
                n330 = In Range and Coerce(upper limit=w737, x=w738, lower limit=w741) -> (In Range?=w740:bool)  [unwired: 1 out]
                n331 = Select(t=0.25 ("Output"), s=w740, f=1.0 ("Output")) -> (s? t:f=w739:dbl)
                n332 = call <vilib>:"CTRE_Phoenix_MotorControl_Set.vi"("Output"=w739, "Control Mode"=w745, "PhoenixMotorControlDevRef"=w747) -> ()  [unwired: 7 in, 2 out]
              }
            }
            n333 = case shown="True" w721 {
              tunnel: "Load Cargo" -> [_ w726]
              tunnel: w716 -> [_ w727]
              frame False {
              }
              frame True {
                w734 = T9 0 items=["PercentOutput"=0, "Position"=1, "Velocity"=2, "Current"=3, "Follower"=5, "MotionProfile"=6, "MotionMagic"=7, "MotionProfileArc"=10, "Disabled"=15] ("Control Mode")
                n334 = call <vilib>:"CTRE_Phoenix_MotorControl_RefNumRegistryGet.vi"("refnum name"="Arm Actuator") -> ("PhoenixMotorControlDevRef"=w736:T2)  [unwired: 9 in, 1 out]
                n335 = Add(x=w726, y=70) -> (x+y=w730:i32)
                n336 = In Range and Coerce(upper limit=w730, x=w727, lower limit=w726) -> (In Range?=w728:bool)  [unwired: 1 out]
                n337 = Select(t=-0.25 ("Output"), s=w728, f=-1.0 ("Output")) -> (s? t:f=w733:dbl)
                n338 = call <vilib>:"CTRE_Phoenix_MotorControl_Set.vi"("Output"=w733, "Control Mode"=w734, "PhoenixMotorControlDevRef"=w736) -> ()  [unwired: 7 in, 2 out]
              }
            }
            n339 = Select(t=T1."Wait", s=w719, f=T1."Load Cargo") -> (s? t:f=w715:T1)
            n340 = call-poly <vilib>:"CTRE_Phoenix_MotorController_Get_Enhanced.vi"("PhoenixMotorControlDevRef"=w717) -> ("AnalogInRaw"=w714:i32)  [unwired: 10 in, 4 out]
          }
          frame "Pre Climb 2" {
            # "Change to \"Climb 2\" after testing"
            # "Actual Position"
            # "Desired Position"
            # "Below"
            # "Neutral"
            # "Above"
            n341 = Add(x="Pre Climb 2", y=20) -> (x+y=w759:i32)
            n342 = Subtract(x="Pre Climb 2", y=20) -> (x-y=w760:i32)
            n343 = In Range and Coerce(upper limit=w759, x=w751, lower limit=w760) -> (In Range?=w755:bool)  [unwired: 1 out]
            n344 = Less?(x="Pre Climb 2", y=w751) -> (x < y?=w757:bool)
            n345 = Greater?(x="Pre Climb 2", y=w751) -> (0:w756:bool)
            n346 = case shown="True" w756 {
              tunnel: "Pre Climb 2" -> [_ w773]
              tunnel: w751 -> [_ w774]
              frame False {
              }
              frame True {
                w781 = T9 0 items=["PercentOutput"=0, "Position"=1, "Velocity"=2, "Current"=3, "Follower"=5, "MotionProfile"=6, "MotionMagic"=7, "MotionProfileArc"=10, "Disabled"=15] ("Control Mode")
                n347 = call <vilib>:"CTRE_Phoenix_MotorControl_RefNumRegistryGet.vi"("refnum name"="Arm Actuator") -> ("PhoenixMotorControlDevRef"=w783:T2)  [unwired: 9 in, 1 out]
                n348 = Subtract(x=w773, y=50) -> (x-y=w777:i32)
                n349 = In Range and Coerce(upper limit=w773, x=w774, lower limit=w777) -> (In Range?=w776:bool)  [unwired: 1 out]
                n350 = Select(t=0.25 ("Output"), s=w776, f=0.5 ("Output")) -> (s? t:f=w775:dbl)
                n351 = call <vilib>:"CTRE_Phoenix_MotorControl_Set.vi"("Output"=w775, "Control Mode"=w781, "PhoenixMotorControlDevRef"=w783) -> ()  [unwired: 7 in, 2 out]
              }
            }
            n352 = case shown="True" w757 {
              tunnel: "Pre Climb 2" -> [_ w762]
              tunnel: w751 -> [_ w763]
              frame False {
              }
              frame True {
                w770 = T9 0 items=["PercentOutput"=0, "Position"=1, "Velocity"=2, "Current"=3, "Follower"=5, "MotionProfile"=6, "MotionMagic"=7, "MotionProfileArc"=10, "Disabled"=15] ("Control Mode")
                n353 = call <vilib>:"CTRE_Phoenix_MotorControl_RefNumRegistryGet.vi"("refnum name"="Arm Actuator") -> ("PhoenixMotorControlDevRef"=w772:T2)  [unwired: 9 in, 1 out]
                n354 = Add(x=w762, y=50) -> (x+y=w766:i32)
                n355 = In Range and Coerce(upper limit=w766, x=w763, lower limit=w762) -> (In Range?=w764:bool)  [unwired: 1 out]
                n356 = Select(t=-0.25 ("Output"), s=w764, f=-0.5 ("Output")) -> (s? t:f=w769:dbl)
                n357 = call <vilib>:"CTRE_Phoenix_MotorControl_Set.vi"("Output"=w769, "Control Mode"=w770, "PhoenixMotorControlDevRef"=w772) -> ()  [unwired: 7 in, 2 out]
              }
            }
            n358 = Select(t=T1."Upward Travel 2", s=w755, f=T1."Pre Climb 2") -> (s? t:f=w749:T1)
            n359 = call-poly <vilib>:"CTRE_Phoenix_MotorController_Get_Enhanced.vi"("PhoenixMotorControlDevRef"=w750) -> ("AnalogInRaw"=w748:i32)  [unwired: 10 in, 4 out]
          }
          frame "Upward Travel 2" {
            # "Uses the arm and jack to climb the habitat's side"
            # "593"
            n360 = for {
              N: 257 -> [_]
              tunnel: w791 -> [w799]
              tunnel: w790 -> [w806]
              tunnel: w789 -> [w805]
              tunnel: [w800] -> w792
              tunnel: "Arm speed-2" -> [w797]
              tunnel: "Jack speed 1-2" -> [w796]
              w802 = T9 0 items=["PercentOutput"=0, "Position"=1, "Velocity"=2, "Current"=3, "Follower"=5, "MotionProfile"=6, "MotionMagic"=7, "MotionProfileArc"=10, "Disabled"=15] ("Control Mode")
              w803 = T9 0 items=["PercentOutput"=0, "Position"=1, "Velocity"=2, "Current"=3, "Follower"=5, "MotionProfile"=6, "MotionMagic"=7, "MotionProfileArc"=10, "Disabled"=15] ("Control Mode")
              w804 = T9 0 items=["PercentOutput"=0, "Position"=1, "Velocity"=2, "Current"=3, "Follower"=5, "MotionProfile"=6, "MotionMagic"=7, "MotionProfileArc"=10, "Disabled"=15] ("Control Mode")
              n361 = call <vilib>:"CTRE_Phoenix_MotorControl_Set.vi"("Output"=w797, "Control Mode"=w803, "PhoenixMotorControlDevRef"=w799) -> ()  [unwired: 7 in, 2 out]
              n362 = call <vilib>:"CTRE_Phoenix_MotorControl_Set.vi"("Output"=w796, "Control Mode"=w804, "PhoenixMotorControlDevRef"=w806) -> ()  [unwired: 7 in, 2 out]
              n363 = call <vilib>:"CTRE_Phoenix_MotorControl_Set.vi"("Output"=0.0, "Control Mode"=w802, "PhoenixMotorControlDevRef"=w805) -> ("PhoenixMotorControlDevRef"=w800:T2)  [unwired: 7 in, 1 out]
              n364 = Wait (ms)(milliseconds to wait=u32 10) -> ()  [unwired: 1 out]
            }
            n365 = for {
              N: 1 -> [_]
              tunnel: [T1."Extra Jack Time 2"] -> w784
              tunnel: w792 -> [_]
              n366 = Wait (ms)(milliseconds to wait=u32 10) -> ()  [unwired: 1 out]
            }
          }
          frame "Extra Jack Time 2" {
            # "extra time given to jack the back end up to get more clearance on the platform"
            # "We may use this"
            n367 = for {
              N: 356 -> [_]
              tunnel: w813 -> [w828]
              tunnel: w812 -> [w827]
              tunnel: w811 -> [w826]
              tunnel: [w820] -> w814
              tunnel: "Jack speed 2-2" -> [w818]
              w823 = T9 0 items=["PercentOutput"=0, "Position"=1, "Velocity"=2, "Current"=3, "Follower"=5, "MotionProfile"=6, "MotionMagic"=7, "MotionProfileArc"=10, "Disabled"=15] ("Control Mode")
              w824 = T9 0 items=["PercentOutput"=0, "Position"=1, "Velocity"=2, "Current"=3, "Follower"=5, "MotionProfile"=6, "MotionMagic"=7, "MotionProfileArc"=10, "Disabled"=15] ("Control Mode")
              w825 = T9 0 items=["PercentOutput"=0, "Position"=1, "Velocity"=2, "Current"=3, "Follower"=5, "MotionProfile"=6, "MotionMagic"=7, "MotionProfileArc"=10, "Disabled"=15] ("Control Mode")
              n368 = call <vilib>:"CTRE_Phoenix_MotorControl_Set.vi"("Output"=0.0, "Control Mode"=w824, "PhoenixMotorControlDevRef"=w828) -> ()  [unwired: 7 in, 2 out]
              n369 = call <vilib>:"CTRE_Phoenix_MotorControl_Set.vi"("Output"=w818, "Control Mode"=w825, "PhoenixMotorControlDevRef"=w827) -> ()  [unwired: 7 in, 2 out]
              n370 = call <vilib>:"CTRE_Phoenix_MotorControl_Set.vi"("Output"=0.0, "Control Mode"=w823, "PhoenixMotorControlDevRef"=w826) -> ("PhoenixMotorControlDevRef"=w820:T2)  [unwired: 7 in, 1 out]
              n371 = Wait (ms)(milliseconds to wait=u32 10) -> ()  [unwired: 1 out]
            }
            n372 = for {
              N: 1 -> [_]
              tunnel: [T1."Forward Travel 2"] -> w807
              tunnel: w814 -> [_]
              n373 = Wait (ms)(milliseconds to wait=u32 10) -> ()  [unwired: 1 out]
            }
          }
          frame "Forward Travel 2" {
            # "Bring the robot forward onto the platform by running the jack foot"
            n374 = for {
              N: 230 -> [_]
              tunnel: w836 -> [w855]
              tunnel: w835 -> [w854]
              tunnel: w834 -> [w853]
              tunnel: [w846] -> w837
              tunnel: "Jack drive 1-2" -> [w845]
              tunnel: w829 -> [w844]
              w850 = T9 0 items=["PercentOutput"=0, "Position"=1, "Velocity"=2, "Current"=3, "Follower"=5, "MotionProfile"=6, "MotionMagic"=7, "MotionProfileArc"=10, "Disabled"=15] ("Control Mode")
              w851 = T9 0 items=["PercentOutput"=0, "Position"=1, "Velocity"=2, "Current"=3, "Follower"=5, "MotionProfile"=6, "MotionMagic"=7, "MotionProfileArc"=10, "Disabled"=15] ("Control Mode")
              w852 = T9 0 items=["PercentOutput"=0, "Position"=1, "Velocity"=2, "Current"=3, "Follower"=5, "MotionProfile"=6, "MotionMagic"=7, "MotionProfileArc"=10, "Disabled"=15] ("Control Mode")
              n375 = call <vilib>:"CTRE_Phoenix_MotorControl_Set.vi"("Output"=0.0, "Control Mode"=w851, "PhoenixMotorControlDevRef"=w855) -> ()  [unwired: 7 in, 2 out]
              n376 = call <vilib>:"CTRE_Phoenix_MotorControl_Set.vi"("Output"=0.0, "Control Mode"=w852, "PhoenixMotorControlDevRef"=w854) -> ()  [unwired: 7 in, 2 out]
              n377 = call <vilib>:"CTRE_Phoenix_MotorControl_Set.vi"("Output"=w845, "Control Mode"=w850, "PhoenixMotorControlDevRef"=w853) -> ("PhoenixMotorControlDevRef"=w846:T2)  [unwired: 7 in, 1 out]
              n378 = call-poly <vilib>:"WPI_RobotDriveHolonomicDrive.vi"("Rotation"=0.0, "Y"=-0.05, "X"=0.0, "RobotDriveDevRef"=w844) -> ()  [unwired: 5 in, 3 out]
              n379 = Wait (ms)(milliseconds to wait=u32 10) -> ()  [unwired: 1 out]
            }
            n380 = for {
              N: 1 -> [_]
              tunnel: [T1."Jack Retrieval 2"] -> w830
              tunnel: w837 -> [_]
              n381 = Wait (ms)(milliseconds to wait=u32 10) -> ()  [unwired: 1 out]
            }
          }
          frame "Jack Retrieval 2" {
            # "bring the jack back up into the robot so we can be completely supported by the hab platform"
            # "This only needs to go up\nfor very little time"
            n382 = for {
              N: 50 -> [_]
              tunnel: w862 -> [w877]
              tunnel: w861 -> [w876]
              tunnel: w860 -> [w875]
              tunnel: [w869] -> w863
              tunnel: "Jack speed 3-2" -> [w867]
              w872 = T9 0 items=["PercentOutput"=0, "Position"=1, "Velocity"=2, "Current"=3, "Follower"=5, "MotionProfile"=6, "MotionMagic"=7, "MotionProfileArc"=10, "Disabled"=15] ("Control Mode")
              w873 = T9 0 items=["PercentOutput"=0, "Position"=1, "Velocity"=2, "Current"=3, "Follower"=5, "MotionProfile"=6, "MotionMagic"=7, "MotionProfileArc"=10, "Disabled"=15] ("Control Mode")
              w874 = T9 0 items=["PercentOutput"=0, "Position"=1, "Velocity"=2, "Current"=3, "Follower"=5, "MotionProfile"=6, "MotionMagic"=7, "MotionProfileArc"=10, "Disabled"=15] ("Control Mode")
              n383 = call <vilib>:"CTRE_Phoenix_MotorControl_Set.vi"("Output"=0.0, "Control Mode"=w873, "PhoenixMotorControlDevRef"=w877) -> ()  [unwired: 7 in, 2 out]
              n384 = call <vilib>:"CTRE_Phoenix_MotorControl_Set.vi"("Output"=w867, "Control Mode"=w874, "PhoenixMotorControlDevRef"=w876) -> ()  [unwired: 7 in, 2 out]
              n385 = call <vilib>:"CTRE_Phoenix_MotorControl_Set.vi"("Output"=0.0, "Control Mode"=w872, "PhoenixMotorControlDevRef"=w875) -> ("PhoenixMotorControlDevRef"=w869:T2)  [unwired: 7 in, 1 out]
              n386 = Wait (ms)(milliseconds to wait=u32 10) -> ()  [unwired: 1 out]
            }
            n387 = for {
              N: 1 -> [_]
              tunnel: w863 -> [_]
              tunnel: [T1."Wait"] -> w856
              n388 = Wait (ms)(milliseconds to wait=u32 10) -> ()  [unwired: 1 out]
            }
          }
        }
      }
    }
  }
  n389 = disable-structure shown="Disabled" {
    frame Disabled {
      n390 = case shown="True" {
        selector: _ -> [_ _]
        tunnel: [w878 w906] -> _
        tunnel: _ -> [w878 _]
        frame False {
        }
        frame True {
          # "wait"
          # "Run the jack in the opposite direction\nto bring it into the robot and to allow \nforward movement all the way onto the platform"
          # "wait"
          # "Give power to jack foot to bring\nthe robot forward onto the platform"
          # "wait"
          # "Bring the back end of the robot\nfarther up, so it is safer to drive forward"
          # "Let the jack down and a little\npower for the arm to maintain level"
          # "98 Position for arm to go to"
          n391 = for {
            N: 50 -> [_]
            tunnel: _ -> [w919]
            tunnel: _ -> [w918]
            tunnel: _ -> [w917]
            tunnel: [w910] -> w879
            tunnel: [w909] -> w880
            tunnel: [w908] -> w881
            w913 = T9 0 items=["PercentOutput"=0, "Position"=1, "Velocity"=2, "Current"=3, "Follower"=5, "MotionProfile"=6, "MotionMagic"=7, "MotionProfileArc"=10, "Disabled"=15] ("Control Mode")
            w915 = T9 0 items=["PercentOutput"=0, "Position"=1, "Velocity"=2, "Current"=3, "Follower"=5, "MotionProfile"=6, "MotionMagic"=7, "MotionProfileArc"=10, "Disabled"=15] ("Control Mode")
            w916 = T9 0 items=["PercentOutput"=0, "Position"=1, "Velocity"=2, "Current"=3, "Follower"=5, "MotionProfile"=6, "MotionMagic"=7, "MotionProfileArc"=10, "Disabled"=15] ("Control Mode")
            n392 = Wait (ms)(milliseconds to wait=u32 10) -> ()  [unwired: 1 out]
            n393 = call <vilib>:"CTRE_Phoenix_MotorControl_Set.vi"("Output"=0.0, "Control Mode"=w913, "PhoenixMotorControlDevRef"=w918) -> ("PhoenixMotorControlDevRef"=w908:T2)  [unwired: 7 in, 1 out]
            n394 = call <vilib>:"CTRE_Phoenix_MotorControl_Set.vi"("Output"=0.0, "Control Mode"=w915, "PhoenixMotorControlDevRef"=w919) -> ("PhoenixMotorControlDevRef"=w909:T2)  [unwired: 7 in, 1 out]
            n395 = call <vilib>:"CTRE_Phoenix_MotorControl_Set.vi"("Output"=0.0, "Control Mode"=w916, "PhoenixMotorControlDevRef"=w917) -> ("PhoenixMotorControlDevRef"=w910:T2)  [unwired: 7 in, 1 out]
          }
          n396 = for {
            N: 116 -> [_]
            tunnel: w879 -> [w991]
            tunnel: w880 -> [w990]
            tunnel: [w989] -> w905
            tunnel: [w985] -> w903
            tunnel: w881 -> [w984]
            tunnel: [w982] -> w902
            w986 = T9 0 items=["PercentOutput"=0, "Position"=1, "Velocity"=2, "Current"=3, "Follower"=5, "MotionProfile"=6, "MotionMagic"=7, "MotionProfileArc"=10, "Disabled"=15] ("Control Mode")
            w987 = T9 0 items=["PercentOutput"=0, "Position"=1, "Velocity"=2, "Current"=3, "Follower"=5, "MotionProfile"=6, "MotionMagic"=7, "MotionProfileArc"=10, "Disabled"=15] ("Control Mode")
            w988 = T9 0 items=["PercentOutput"=0, "Position"=1, "Velocity"=2, "Current"=3, "Follower"=5, "MotionProfile"=6, "MotionMagic"=7, "MotionProfileArc"=10, "Disabled"=15] ("Control Mode")
            n397 = Wait (ms)(milliseconds to wait=u32 10) -> ()  [unwired: 1 out]
            n398 = call <vilib>:"CTRE_Phoenix_MotorControl_Set.vi"("Control Mode"=w987, "PhoenixMotorControlDevRef"=w990) -> ("PhoenixMotorControlDevRef"=w989:T2)  [unwired: 8 in, 1 out]
            n399 = call <vilib>:"CTRE_Phoenix_MotorControl_Set.vi"("Control Mode"=w988, "PhoenixMotorControlDevRef"=w991) -> ("PhoenixMotorControlDevRef"=w985:T2)  [unwired: 8 in, 1 out]
            n400 = call <vilib>:"CTRE_Phoenix_MotorControl_Set.vi"("Output"=0.0, "Control Mode"=w986, "PhoenixMotorControlDevRef"=w984) -> ("PhoenixMotorControlDevRef"=w982:T2)  [unwired: 7 in, 1 out]
          }
          n401 = for {
            N: 217 -> [_]
            tunnel: w905 -> [w979]
            tunnel: [w978] -> w904
            tunnel: w903 -> [w974]
            tunnel: w902 -> [w972]
            tunnel: [w970] -> w901
            tunnel: [w969] -> w900
            w975 = T9 0 items=["PercentOutput"=0, "Position"=1, "Velocity"=2, "Current"=3, "Follower"=5, "MotionProfile"=6, "MotionMagic"=7, "MotionProfileArc"=10, "Disabled"=15] ("Control Mode")
            w976 = T9 0 items=["PercentOutput"=0, "Position"=1, "Velocity"=2, "Current"=3, "Follower"=5, "MotionProfile"=6, "MotionMagic"=7, "MotionProfileArc"=10, "Disabled"=15] ("Control Mode")
            w977 = T9 0 items=["PercentOutput"=0, "Position"=1, "Velocity"=2, "Current"=3, "Follower"=5, "MotionProfile"=6, "MotionMagic"=7, "MotionProfileArc"=10, "Disabled"=15] ("Control Mode")
            n402 = Wait (ms)(milliseconds to wait=u32 10) -> ()  [unwired: 1 out]
            n403 = call <vilib>:"CTRE_Phoenix_MotorControl_Set.vi"("Control Mode"=w975, "PhoenixMotorControlDevRef"=w979) -> ("PhoenixMotorControlDevRef"=w978:T2)  [unwired: 8 in, 1 out]
            n404 = call <vilib>:"CTRE_Phoenix_MotorControl_Set.vi"("Output"=0.0, "Control Mode"=w976, "PhoenixMotorControlDevRef"=w972) -> ("PhoenixMotorControlDevRef"=w970:T2)  [unwired: 7 in, 1 out]
            n405 = call <vilib>:"CTRE_Phoenix_MotorControl_Set.vi"("Output"=0.0, "Control Mode"=w977, "PhoenixMotorControlDevRef"=w974) -> ("PhoenixMotorControlDevRef"=w969:T2)  [unwired: 7 in, 1 out]
          }
          n406 = for {
            N: 40 -> [_]
            tunnel: w904 -> [w967]
            tunnel: w901 -> [w966]
            tunnel: w900 -> [w965]
            tunnel: [w958] -> w899
            tunnel: [w957] -> w898
            tunnel: [w956] -> w897
            w961 = T9 0 items=["PercentOutput"=0, "Position"=1, "Velocity"=2, "Current"=3, "Follower"=5, "MotionProfile"=6, "MotionMagic"=7, "MotionProfileArc"=10, "Disabled"=15] ("Control Mode")
            w963 = T9 0 items=["PercentOutput"=0, "Position"=1, "Velocity"=2, "Current"=3, "Follower"=5, "MotionProfile"=6, "MotionMagic"=7, "MotionProfileArc"=10, "Disabled"=15] ("Control Mode")
            w964 = T9 0 items=["PercentOutput"=0, "Position"=1, "Velocity"=2, "Current"=3, "Follower"=5, "MotionProfile"=6, "MotionMagic"=7, "MotionProfileArc"=10, "Disabled"=15] ("Control Mode")
            n407 = Wait (ms)(milliseconds to wait=u32 10) -> ()  [unwired: 1 out]
            n408 = call <vilib>:"CTRE_Phoenix_MotorControl_Set.vi"("Output"=0.0, "Control Mode"=w961, "PhoenixMotorControlDevRef"=w966) -> ("PhoenixMotorControlDevRef"=w956:T2)  [unwired: 7 in, 1 out]
            n409 = call <vilib>:"CTRE_Phoenix_MotorControl_Set.vi"("Output"=0.0, "Control Mode"=w963, "PhoenixMotorControlDevRef"=w967) -> ("PhoenixMotorControlDevRef"=w957:T2)  [unwired: 7 in, 1 out]
            n410 = call <vilib>:"CTRE_Phoenix_MotorControl_Set.vi"("Output"=0.0, "Control Mode"=w964, "PhoenixMotorControlDevRef"=w965) -> ("PhoenixMotorControlDevRef"=w958:T2)  [unwired: 7 in, 1 out]
          }
          n411 = for {
            N: 230 -> [_]
            tunnel: w899 -> [w951]
            tunnel: w898 -> [w950]
            tunnel: w897 -> [w949]
            tunnel: [w946] -> w896
            tunnel: [w945] -> w895
            tunnel: [w944] -> w894
            w952 = T9 0 items=["PercentOutput"=0, "Position"=1, "Velocity"=2, "Current"=3, "Follower"=5, "MotionProfile"=6, "MotionMagic"=7, "MotionProfileArc"=10, "Disabled"=15] ("Control Mode")
            w953 = T9 0 items=["PercentOutput"=0, "Position"=1, "Velocity"=2, "Current"=3, "Follower"=5, "MotionProfile"=6, "MotionMagic"=7, "MotionProfileArc"=10, "Disabled"=15] ("Control Mode")
            w954 = T9 0 items=["PercentOutput"=0, "Position"=1, "Velocity"=2, "Current"=3, "Follower"=5, "MotionProfile"=6, "MotionMagic"=7, "MotionProfileArc"=10, "Disabled"=15] ("Control Mode")
            n412 = Wait (ms)(milliseconds to wait=u32 10) -> ()  [unwired: 1 out]
            n413 = call <vilib>:"CTRE_Phoenix_MotorControl_Set.vi"("Control Mode"=w952, "PhoenixMotorControlDevRef"=w949) -> ("PhoenixMotorControlDevRef"=w944:T2)  [unwired: 8 in, 1 out]
            n414 = call <vilib>:"CTRE_Phoenix_MotorControl_Set.vi"("Output"=0.0, "Control Mode"=w953, "PhoenixMotorControlDevRef"=w950) -> ("PhoenixMotorControlDevRef"=w945:T2)  [unwired: 7 in, 1 out]
            n415 = call <vilib>:"CTRE_Phoenix_MotorControl_Set.vi"("Output"=0.0, "Control Mode"=w954, "PhoenixMotorControlDevRef"=w951) -> ("PhoenixMotorControlDevRef"=w946:T2)  [unwired: 7 in, 1 out]
          }
          n416 = for {
            N: 80 -> [_]
            tunnel: w896 -> [w939]
            tunnel: w895 -> [w938]
            tunnel: w894 -> [w937]
            tunnel: [w933] -> w893
            tunnel: [w932] -> w892
            tunnel: [w931] -> w891
            w940 = T9 0 items=["PercentOutput"=0, "Position"=1, "Velocity"=2, "Current"=3, "Follower"=5, "MotionProfile"=6, "MotionMagic"=7, "MotionProfileArc"=10, "Disabled"=15] ("Control Mode")
            w941 = T9 0 items=["PercentOutput"=0, "Position"=1, "Velocity"=2, "Current"=3, "Follower"=5, "MotionProfile"=6, "MotionMagic"=7, "MotionProfileArc"=10, "Disabled"=15] ("Control Mode")
            w942 = T9 0 items=["PercentOutput"=0, "Position"=1, "Velocity"=2, "Current"=3, "Follower"=5, "MotionProfile"=6, "MotionMagic"=7, "MotionProfileArc"=10, "Disabled"=15] ("Control Mode")
            n417 = Wait (ms)(milliseconds to wait=u32 10) -> ()  [unwired: 1 out]
            n418 = call <vilib>:"CTRE_Phoenix_MotorControl_Set.vi"("Output"=0.0, "Control Mode"=w940, "PhoenixMotorControlDevRef"=w937) -> ("PhoenixMotorControlDevRef"=w931:T2)  [unwired: 7 in, 1 out]
            n419 = call <vilib>:"CTRE_Phoenix_MotorControl_Set.vi"("Output"=0.0, "Control Mode"=w941, "PhoenixMotorControlDevRef"=w938) -> ("PhoenixMotorControlDevRef"=w933:T2)  [unwired: 7 in, 1 out]
            n420 = call <vilib>:"CTRE_Phoenix_MotorControl_Set.vi"("Output"=0.0, "Control Mode"=w942, "PhoenixMotorControlDevRef"=w939) -> ("PhoenixMotorControlDevRef"=w932:T2)  [unwired: 7 in, 1 out]
          }
          n421 = for {
            N: 325 -> [_]
            tunnel: w893 -> [w928]
            tunnel: w892 -> [w923]
            tunnel: w891 -> [w922]
            tunnel: [w920] -> w884
            w926 = T9 0 items=["PercentOutput"=0, "Position"=1, "Velocity"=2, "Current"=3, "Follower"=5, "MotionProfile"=6, "MotionMagic"=7, "MotionProfileArc"=10, "Disabled"=15] ("Control Mode")
            w927 = T9 0 items=["PercentOutput"=0, "Position"=1, "Velocity"=2, "Current"=3, "Follower"=5, "MotionProfile"=6, "MotionMagic"=7, "MotionProfileArc"=10, "Disabled"=15] ("Control Mode")
            w929 = T9 0 items=["PercentOutput"=0, "Position"=1, "Velocity"=2, "Current"=3, "Follower"=5, "MotionProfile"=6, "MotionMagic"=7, "MotionProfileArc"=10, "Disabled"=15] ("Control Mode")
            n422 = Wait (ms)(milliseconds to wait=u32 10) -> ()  [unwired: 1 out]
            n423 = call <vilib>:"CTRE_Phoenix_MotorControl_Set.vi"("Control Mode"=w929, "PhoenixMotorControlDevRef"=w928) -> ()  [unwired: 8 in, 2 out]
            n424 = call <vilib>:"CTRE_Phoenix_MotorControl_Set.vi"("Output"=0.0, "Control Mode"=w926, "PhoenixMotorControlDevRef"=w922) -> ("PhoenixMotorControlDevRef"=w920:T2)  [unwired: 7 in, 1 out]
            n425 = call <vilib>:"CTRE_Phoenix_MotorControl_Set.vi"("Output"=0.0, "Control Mode"=w927, "PhoenixMotorControlDevRef"=w923) -> ()  [unwired: 7 in, 2 out]
          }
          n426 = for {
            N: 1 -> [_]
            tunnel: [_] -> w906
            tunnel: w884 -> [_]
            # "go to\nwait \ncase"
            n427 = Wait (ms)(milliseconds to wait=u32 10) -> ()  [unwired: 1 out]
          }
        }
      }
    }
    frame Enabled {
    }
  }
